vi "Main.vi"(11 "Module Admin":refnum<class "Delacor_lib_QMH_Cloneable Module Admin.lvclass">) -> ()   [LabVIEW 2020, in "FCR100.lvlib"]
doc: "This template is based off of the Queued Message Handler design pattern and the Queued Message Handler project template that ships with LabVIEW.\n\nThe main difference is that the queue is private to this module and communication between modules is performed via Broadcast and Request events.\n\nRequest events are wrapped in public API methods and are handled in the Event Handling Loop (EHL) of this VI. Any module can register for Broadcast events sent by this module. The EHL generates messages based on user interface actions.\n\nThe Message Handling Loop (MHL) processes messages generated by the EHL, or by other messages. The messages are string values, so new messages can be added easily to the Message Cases case structure in the MHL. Each message cluster can also provide an optional value for Message Data, which is a variant that can be converted to whatever message-specific data is required.\n_____\nBased on DQMH Project Template 6.1.0.94."
uses:
  FCR100.lvlib
  <vilib>/Delacor/Delacor QMH/Libraries/Cloneable Module Admin_class/Delacor_lib_QMH_Cloneable Module Admin.lvclass
  C:/Program Files (x86)/National Instruments/LabVIEW 2020/vi.lib/Delacor/Delacor QMH/Libraries/Module Admin_class/Delacor_lib_QMH_Module Admin.lvclass
  Support/Device state -- enum.ctl
  Support/Device states -- cluster.ctl
  Module Data--cluster.ctl
  Support/Device connection cluster -- cluster.ctl
  Support/HL data -- cluster.ctl
  <vilib>/Delacor/Delacor QMH/Libraries/Message Queue_class/Delacor_lib_QMH_Message Queue.lvclass/Delacor_lib_QMH_Message Queue.ctl
  <vilib>/Delacor/Delacor QMH/Libraries/Cloneable Module Admin_class/Delacor_lib_QMH_Cloneable Module Admin.lvclass/Delacor_lib_QMH_Cloneable Module Admin.ctl
  Stop Argument--cluster.ctl
  Connect with dialog Argument--cluster.ctl
  Connect with dialog (Reply Payload)--cluster.ctl
  Change configuration state Argument--cluster.ctl
  Change disable state Argument--cluster.ctl
  Search Home Argument--cluster.ctl
  Stop movement Argument--cluster.ctl
  Get state Argument--cluster.ctl
  Get state (Reply Payload)--cluster.ctl
  Set acceleration Argument--cluster.ctl
  Get acceleration Argument--cluster.ctl
  Get acceleration (Reply Payload)--cluster.ctl
  Set velocity Argument--cluster.ctl
  Get velocity Argument--cluster.ctl
  Get velocity (Reply Payload)--cluster.ctl
  Get ETA Argument--cluster.ctl
  Get ETA (Reply Payload)--cluster.ctl
  Move absolute Argument--cluster.ctl
  Move relative Argument--cluster.ctl
  Get current position Argument--cluster.ctl
  Get current position (Reply Payload)--cluster.ctl
  <vilib>/Delacor/Delacor QMH/Libraries/Module Admin_class/Delacor_lib_QMH_Module Admin.lvclass/Delacor_lib_QMH_Module Admin.ctl
  Reset controller Argument--cluster.ctl
  Find instruments Argument--cluster.ctl
  Find instruments (Reply Payload)--cluster.ctl
  Connect wihtout dialog Argument--cluster.ctl
  Disconnect Argument--cluster.ctl
  Continuously check state Argument--cluster.ctl
  Stop checking state Argument--cluster.ctl
  Configure simultaneous move Argument--cluster.ctl
  Get simultaneous move config Argument--cluster.ctl
  Get simultaneous move config (Reply Payload)--cluster.ctl
  Execute simultaneous move Argument--cluster.ctl
  <vilib>/Utility/miscctls.llb/LVPointTypeDef.ctl
  <vilib>/Instr/_visa.llb/VISA Flush IO Buffer Mask.ctl
  Support/Wake HL data -- cluster.ctl
  <vilib>/Delacor/Delacor QMH/Libraries/Message Queue_class/Delacor_lib_QMH_Enqueue Message (Array).vi
  <vilib>/Delacor/Delacor QMH/Libraries/Cloneable Module Admin_class/Delacor_lib_QMH_Get Module ID.vi
  <vilib>/Delacor/Delacor QMH/Libraries/Message Queue_class/Delacor_lib_QMH_Enqueue Message (Single).vi
  <vilib>/Delacor/Delacor QMH/Libraries/Module Admin_class/Delacor_lib_QMH_Get External Launch.vi
  <vilib>/Utility/error.llb/Error Cluster From Error Code.vi
  <vilib>/ErrorRing/Error Ring.xnode
  <vilib>/Delacor/Delacor QMH/Libraries/Message Queue_class/Delacor_lib_QMH_Message Queue.lvclass
panel:
  in  "Device state":T1=enum."Configuration"
  out "error out":errorcluster
  out "Status":string
  # "Other QMH Modules communicate with this Module via its Public API (wrappers for its Request Events).\n\nThis Module communicates with other Modules via its Broadcast Events.\nAny module that wants to get these messages, just registers for this module's Broadcast events."
  # "This template is for the Delacor Modified Queued Message Handler design pattern.\n\nSee the block diagram for more information on how to use this template."
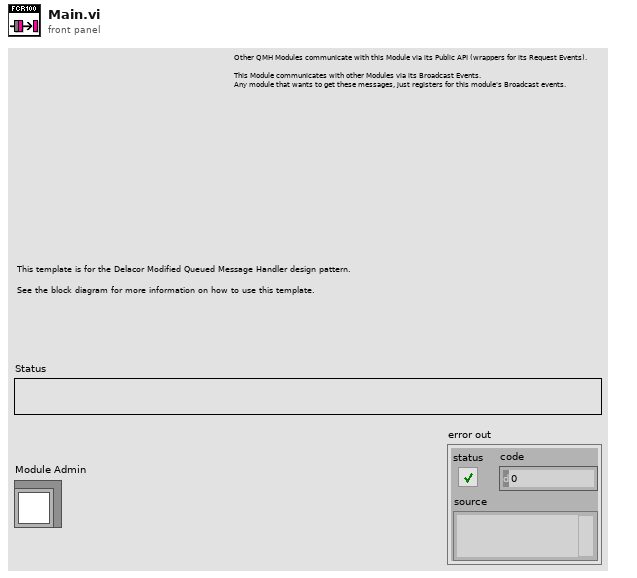
[diagram p1: front panel]
types:
  T1 = typedef "FCR100.lvlib/Device state -- enum.ctl" = enum16{"Not referenced", "Configuration", "Disable", "Ready", "Homing", "Motion"}
  T2 = typedef "FCR100.lvlib/Device states -- cluster.ctl" = cluster{"Address":u8, "Device state out":T1}
  T3 = typedef "FCR100.lvlib/Request Events--cluster.ctl" = cluster{"Stop Module":refnum<user-event>, "Show Panel":refnum<user-event>, "Hide Panel":refnum<user-event>, "Show Diagram":refnum<user-event>, "Get Module Execution Status":refnum<user-event>, "Connect with dialog":refnum<user-event>, "Change configuration state":refnum<user-event>, "Change disable state":refnum<user-event>, "Search Home":refnum<user-event>, "Stop movement":refnum<user-event>, "Get state":refnum<user-event>, "Set acceleration":refnum<user-event>, "Get acceleration":refnum<user-event>, "Set velocity":refnum<user-event>, "Get velocity":refnum<user-event>, "Get ETA":refnum<user-event>, "Move absolute":refnum<user-event>, "Move relative":refnum<user-event>, "Get current position":refnum<user-event>, "Reset controller":refnum<user-event>, "Find instruments":refnum<user-event>, "Connect wihtout dialog":refnum<user-event>, "Disconnect":refnum<user-event>, "Continuously check state":refnum<user-event>, "Stop checking state":refnum<user-event>, "Configure simultaneous move":refnum<user-event>, "Get simultaneous move config":refnum<user-event>, "Execute simultaneous move":refnum<user-event>}
  T4 = cluster{"Wake HL":refnum<user-event>, "Sleep HL":refnum<user-event>}
  T5 = typedef "FCR100.lvlib/HL data -- cluster.ctl" = cluster{"Instrument Channel":string, "Current state":T1, "Desired state":T1, "Address":u8, "Module ID":i32}
  T6 = typedef "FCR100.lvlib/Module Data--cluster.ctl" = cluster{"Status":string, "Device Connection Cluster":T7, "Connected?":bool, "Devices states":T1[], "Instrument Channel":string}
  T7 = typedef "Device connection cluster -- cluster.ctl" = cluster{"VISA resource name":refnum<visa-resource-name>, "Device name":string, "Controller address":i32, "error":errorcluster}
  T8 = enum32{"invalid lock state", "Not Locked", "Locked (No Password)", "Password-protected"}
  T9 = typedef "FCR100.lvlib/Stop Argument--cluster.ctl" = cluster{"Module ID":i32, "Origin":string, "Exit via Stop Module Req?":bool, "Wait for Module to stop?":bool}
  T10 = typedef "FCR100.lvlib/Connect with dialog Argument--cluster.ctl" = cluster{"Module ID":i32, "Baud Rate":u32, "Wait Notifier":refnum<notifier>, "wait for reply":bool}
  T11 = typedef "FCR100.lvlib/Change configuration state Argument--cluster.ctl" = cluster{"Module ID":i32, "Enter/(leave)":bool, "Address":u8}
  T12 = typedef "FCR100.lvlib/Change disable state Argument--cluster.ctl" = cluster{"Module ID":i32, "Enter/Leave":bool, "Address":u8}
  T13 = typedef "FCR100.lvlib/Search Home Argument--cluster.ctl" = cluster{"Module ID":i32, "Address":u8}
  T14 = typedef "FCR100.lvlib/Stop movement Argument--cluster.ctl" = cluster{"Module ID":i32, "Address":u8}
  T15 = typedef "FCR100.lvlib/Get state Argument--cluster.ctl" = cluster{"Module ID":i32, "Address":u8, "Wait Notifier":refnum<notifier>, "wait for reply":bool}
  T16 = typedef "FCR100.lvlib/Set acceleration Argument--cluster.ctl" = cluster{"Module ID":i32, "Address":u8, "Acceleration":u16}
  T17 = typedef "FCR100.lvlib/Get acceleration Argument--cluster.ctl" = cluster{"Module ID":i32, "Address":u8, "Wait Notifier":refnum<notifier>, "wait for reply":bool}
  T18 = typedef "FCR100.lvlib/Set velocity Argument--cluster.ctl" = cluster{"Module ID":i32, "Address":u8, "Velocity":u16}
  T19 = typedef "FCR100.lvlib/Get velocity Argument--cluster.ctl" = cluster{"Module ID":i32, "Address":u8, "Wait Notifier":refnum<notifier>, "wait for reply":bool}
  T20 = typedef "FCR100.lvlib/Get ETA Argument--cluster.ctl" = cluster{"Module ID":i32, "Address":u8, "Position":dbl, "Wait Notifier":refnum<notifier>, "wait for reply":bool}
  T21 = typedef "FCR100.lvlib/Move absolute Argument--cluster.ctl" = cluster{"Module ID":i32, "Address":u8, "Position":dbl}
  T22 = typedef "FCR100.lvlib/Move relative Argument--cluster.ctl" = cluster{"Module ID":i32, "Address":u8, "Position":dbl}
  T23 = typedef "FCR100.lvlib/Get current position Argument--cluster.ctl" = cluster{"Module ID":i32, "Address":u8, "Wait Notifier":refnum<notifier>, "wait for reply":bool}
  T24 = typedef "FCR100.lvlib/Reset controller Argument--cluster.ctl" = cluster{"Module ID":i32, "Address":u8}
  T25 = typedef "FCR100.lvlib/Find instruments Argument--cluster.ctl" = cluster{"Module ID":i32, "Wait Notifier":refnum<notifier>, "wait for reply":bool}
  T26 = typedef "FCR100.lvlib/Connect wihtout dialog Argument--cluster.ctl" = cluster{"Module ID":i32, "VISA resource":refnum<visa-resource-name>, "baud rate":u32}
  T27 = typedef "FCR100.lvlib/Disconnect Argument--cluster.ctl" = cluster{"Module ID":i32, "Boolean":bool}
  T28 = typedef "FCR100.lvlib/Continuously check state Argument--cluster.ctl" = cluster{"Module ID":i32, "Address":u8, "Desired state":T1, "Timeout":i32}
  T29 = typedef "FCR100.lvlib/Stop checking state Argument--cluster.ctl" = cluster{"Module ID":i32, "Address":u8}
  T30 = typedef "FCR100.lvlib/Configure simultaneous move Argument--cluster.ctl" = cluster{"Module ID":i32, "Address":u8, "Position":dbl}
  T31 = typedef "FCR100.lvlib/Get simultaneous move config Argument--cluster.ctl" = cluster{"Module ID":i32, "Address":u8, "Wait Notifier":refnum<notifier>, "wait for reply":bool}
  T32 = typedef "FCR100.lvlib/Execute simultaneous move Argument--cluster.ctl" = cluster{"Module ID":i32, "Boolean":bool}
  T33 = typedef "LVPointTypeDef.ctl" = cluster{"Horizontal":i16, "Vertical":i16}
  T34 = enum32{"Invalid", "Standard", "Closed", "Hidden", "Minimized", "Maximized"}
  T35 = typedef "FCR100.lvlib/Find instruments (Reply Payload)--cluster.ctl" = cluster{"error":errorcluster, "Resource Names":string[], "Interface Names":string[]}
  T36 = typedef "FCR100.lvlib/Connect with dialog (Reply Payload)--cluster.ctl" = cluster{"Connected?":bool, "error":errorcluster}
  T37 = typedef "FCR100.lvlib/Get state (Reply Payload)--cluster.ctl" = cluster{"Device state":T1, "error":errorcluster}
  T38 = typedef "FCR100.lvlib/Get acceleration (Reply Payload)--cluster.ctl" = cluster{"Acceleration":u16, "error":errorcluster}
  T39 = typedef "FCR100.lvlib/Get velocity (Reply Payload)--cluster.ctl" = cluster{"Velocity":u16, "error":errorcluster}
  T40 = typedef "FCR100.lvlib/Get ETA (Reply Payload)--cluster.ctl" = cluster{"ETA":dbl, "error":errorcluster}
  T41 = typedef "FCR100.lvlib/Get current position (Reply Payload)--cluster.ctl" = cluster{"Position":dbl, "error":errorcluster}
  T42 = typedef "FCR100.lvlib/Wake HL data -- cluster.ctl" = cluster{"Timeout":i32, "Instrument Channel":string, "Address":u8, "Current state":T1, "Desired state":T1, "Module ID":i32}
  T43 = typedef "FCR100.lvlib/Get simultaneous move config (Reply Payload)--cluster.ctl" = cluster{"Response":string, "error":errorcluster}
  T44 = cluster{"VISA resource name":refnum<visa-resource-name>, "Device name":string, "Controller address":i32, "error":errorcluster}
  T45 = typedef "VISA Flush IO Buffer Mask.ctl" = u16
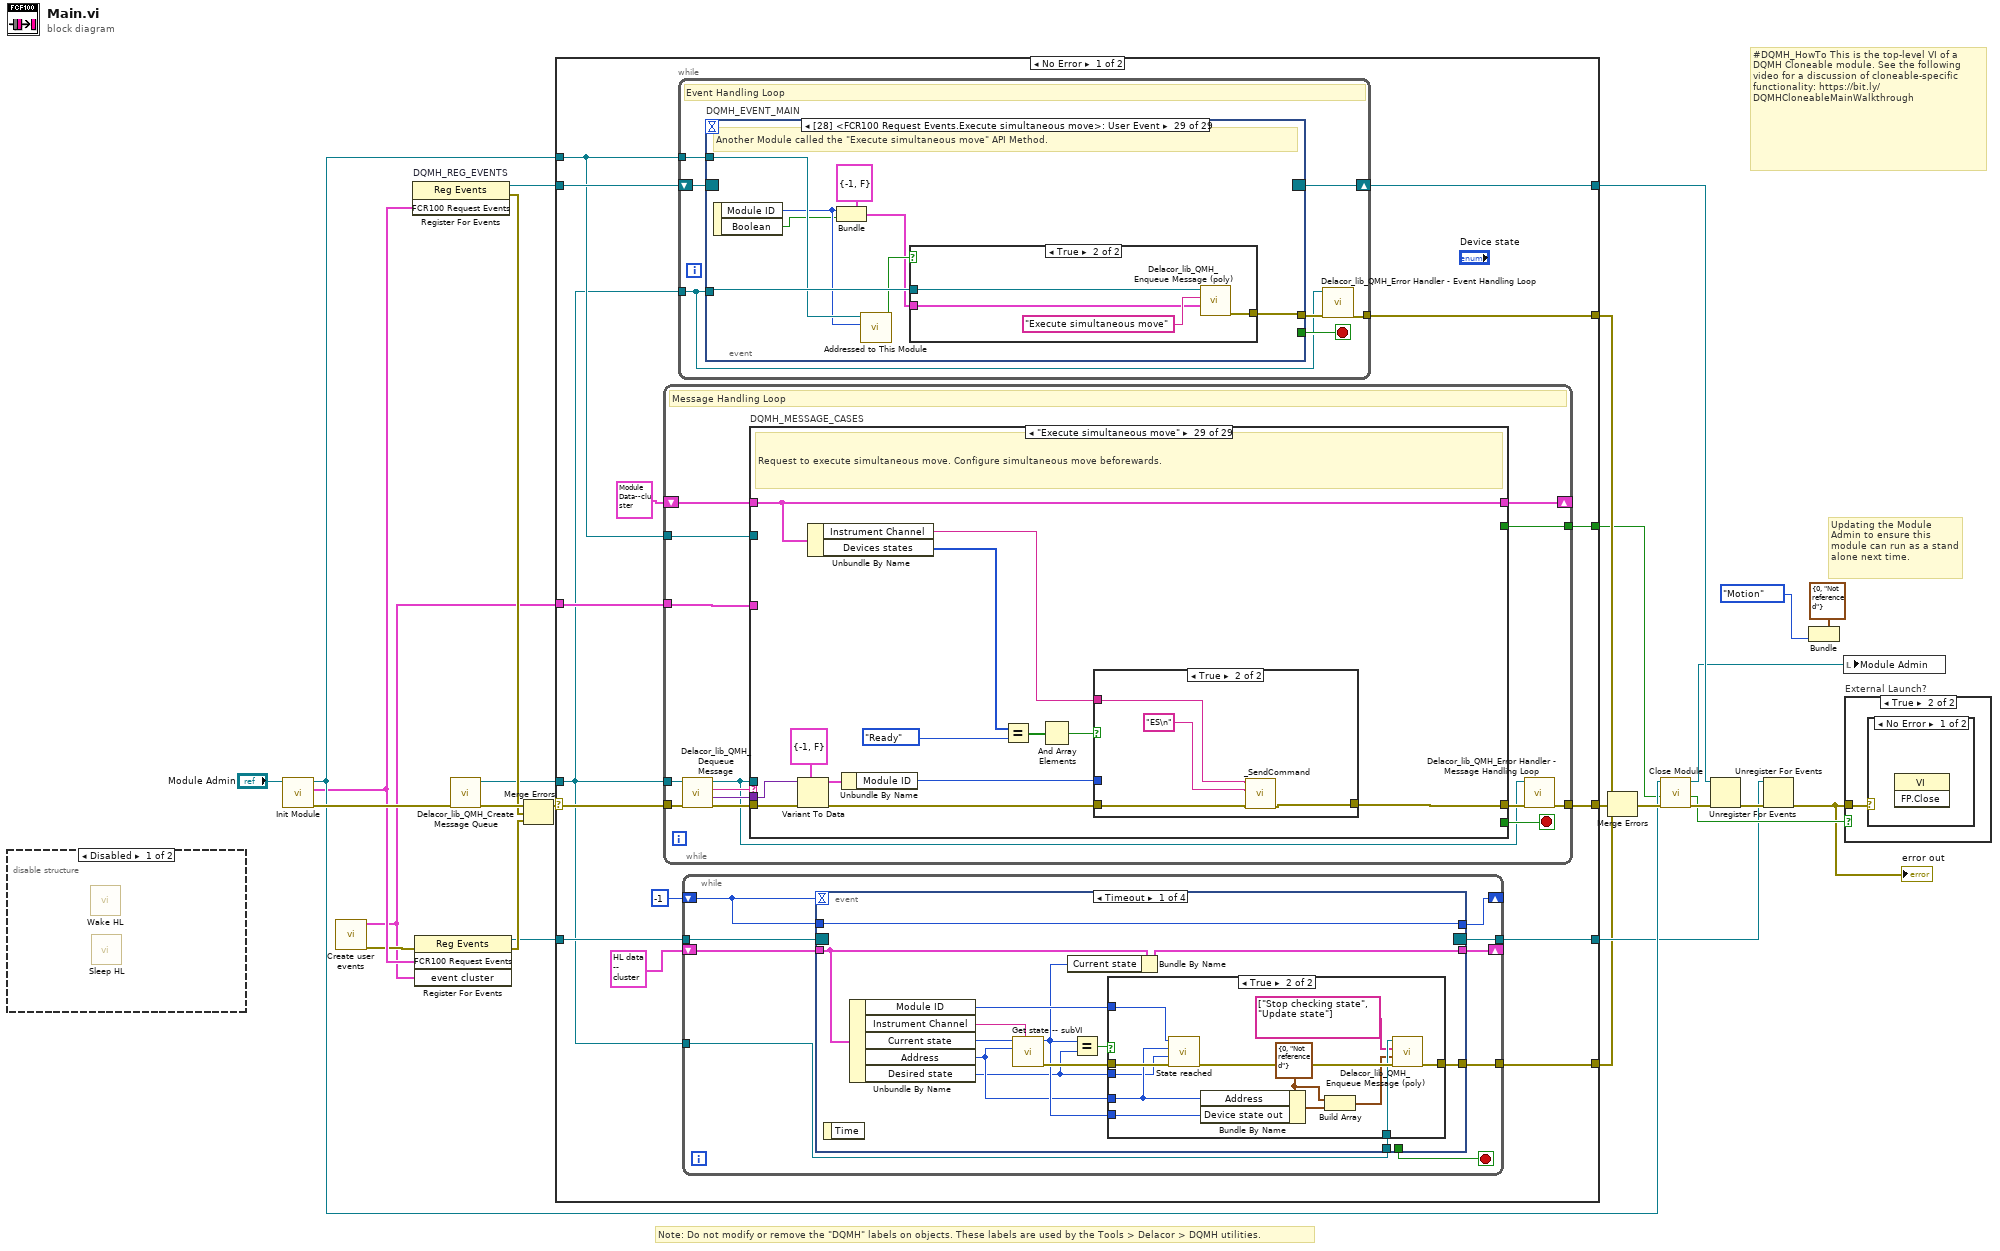
[diagram p0: block diagram]
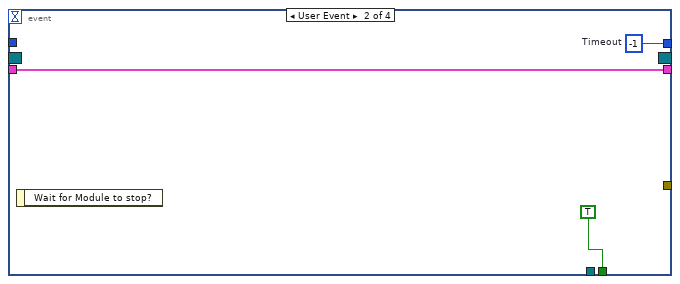
[diagram p4: hidden frame]
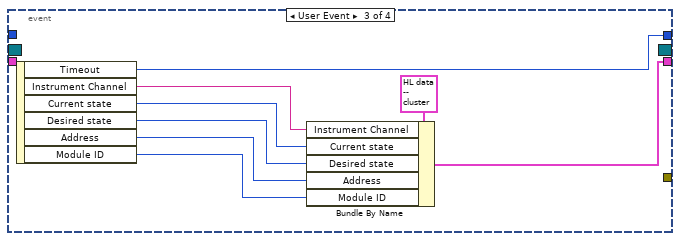
[diagram p5: hidden frame]
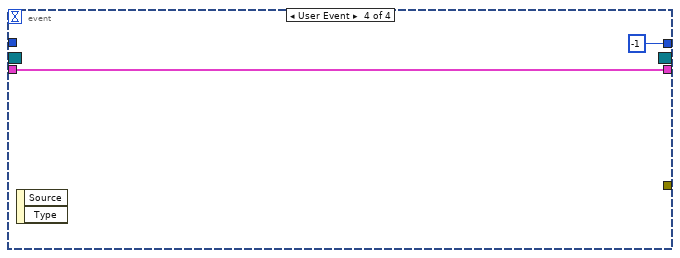
[diagram p6: hidden frame]
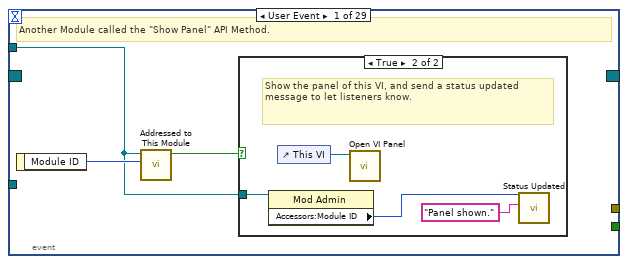
[diagram p7: hidden frame]
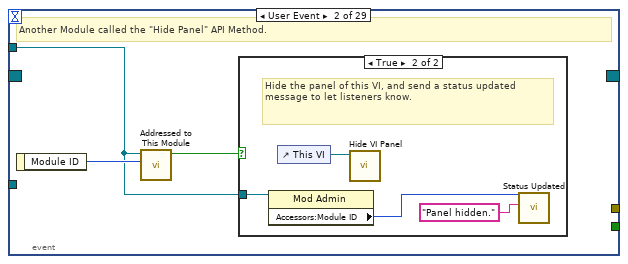
[diagram p9: hidden frame]
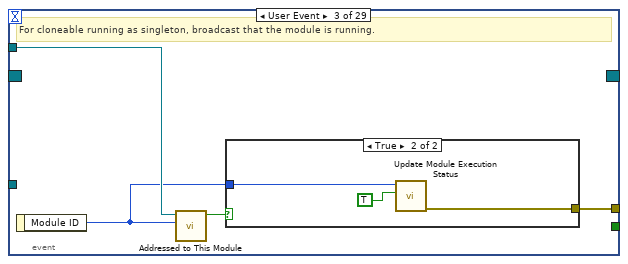
[diagram p11: hidden frame]
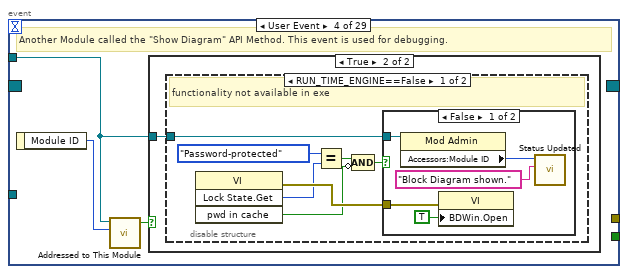
[diagram p13: hidden frame]
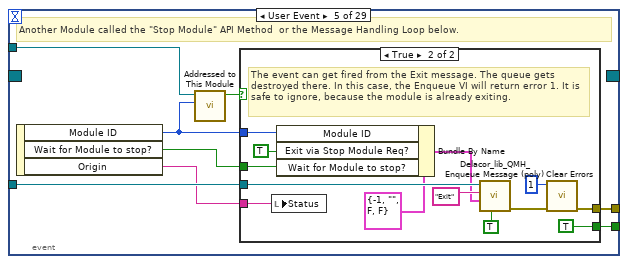
[diagram p17: hidden frame]
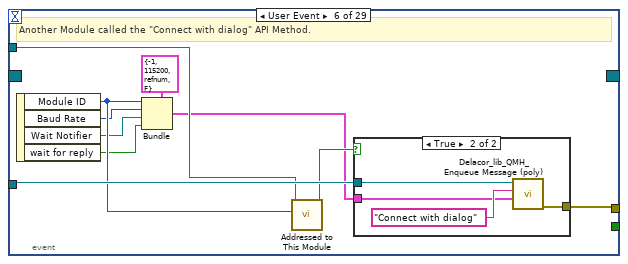
[diagram p19: hidden frame]
diagram:
  # "#DQMH_HowTo This is the top-level VI of a DQMH Cloneable module. See the following video for a discussion of cloneable-specific functionality: https://bit.ly/DQMHCloneableMainWalkthrough"
  # "Note: Do not modify or remove the \"DQMH\" labels on objects. These labels are used by the Tools > Delacor > DQMH utilities."
  # "Updating the Module Admin to ensure this module can run as a stand alone next time."
  n1 = disable-structure shown="Disabled" {
    frame Disabled {
      n2 = call "Wake HL.vi"() -> ()  [unwired: 11 in, 1 out]
      n3 = call "Sleep HL.vi"() -> ()  [unwired: 11 in, 1 out]
    }
    frame Enabled {
    }
  }
  n4 = call "Init Module.vi"("Cloneable Module Admin in"="Module Admin") -> ("error out"=w24:errorcluster, "FCR100 Request Events"=w11:T3, "Cloneable Module Admin out"=w15:refnum<class "Delacor_lib_QMH_Cloneable Module Admin.lvclass">)  [unwired: 8 in]
  n5 = call "Create user events.vi"() -> ("error out"=w10:errorcluster, "event cluster"=w7:T4)  [unwired: 10 in]
  n6 = register-events "DQMH_REG_EVENTS"(w11) -> (reference out=w18:refnum<event-registration>, error out=w20:errorcluster)  [unwired: 2 in]
  n7 = register-events(error in=w10, w11, w7) -> (reference out=w8:refnum<event-registration>, error out=w9:errorcluster)  [unwired: 1 in]
  n8 = call <vilib>:"Delacor_lib_QMH_Create Message Queue.vi"("error in"=w24) -> ("error out"=w22:errorcluster, "Message Queue"=w17:refnum<class "Delacor_lib_QMH_Message Queue.lvclass">)  [unwired: 9 in]
  n9 = Merge Errors(w22, w20, w9) -> (w21:errorcluster)
  n10 = case shown="No Error" w21 {
    selector: w21 -> [w40 w1397]
    tunnel: [w42 w1396] -> w25
    tunnel: [w39 w1404] -> w19
    tunnel: w18 -> [w37 w1404]
    tunnel: w17 -> [w31 w1395]
    tunnel: [w41 _] -> w26
    tunnel: w15 -> [w36 w1400]
    tunnel: [w35 _] -> w13
    tunnel: w8 -> [w34 w1394]
    tunnel: w7 -> [w33 _]
    tunnel: [w32 w1394] -> w4
    tunnel: [w28 _] -> w3
    frame No Error {
      n11 = while {
        tunnel: w31 -> [w471]
        shift-right: [w475] -> _
        shift-left: T6 {"Status"="", "Device Connection Cluster"={"VISA resource name"="", "Device name"="", "Controller address"=0, "error"={"status"=FALSE, "code"=0, "source"=""}}, "Connected?"=FALSE, "Devices states"=[], "Instrument Channel"="GPIB/0:4,0"} ("Data Cluster") -> [w476]
        tunnel: w40 -> [w479]
        tunnel: [w477] -> w42
        tunnel: w36 -> [w469]
        tunnel: [w468] -> w35
        tunnel: w33 -> [w467]
        stop <- w474 stop-if-true
        # "Message Handling Loop"
        n12 = call-dynamic "Delacor_lib_QMH_Dequeue Message.vi"("error in"=w479, "Message Queue in"=w471) -> ("error out"=w478:errorcluster, "Message Data"=w472:variant, "Message"=w473:string, "Message Queue out"=w470:refnum<class "Delacor_lib_QMH_Message Queue.lvclass">)  [unwired: 6 in]
        n13 = case "DQMH_MESSAGE_CASES" shown="\"Execute simultaneous move\"" w473 {
          selector: w473 -> [_ _ _ _ _ _ _ _ _ _ _ _ _ _ _ _ _ _ _ _ _ _ _ w1258 _ _ _ _ _]
          tunnel: w470 -> [_ _ _ _ _ _ w661 w707 w746 w792 w834 _ _ _ _ _ w1066 w1115 _ _ _ w1223 w1248 _ _ _ _ _ _]
          tunnel: w478 -> [w499 w515 w530 w605 w639 w651 w669 w715 w755 w800 w846 w864 w906 w945 w987 w1031 w1077 w1126 w1176 w1204 w1221 w1232 w1254 w1260 w1287 w1296 w1310 w1348 w1385]
          tunnel: [w497 w505 w520 w596 w627 w649 w663 w710 w750 w794 w837 w859 w897 w939 w978 w1022 w1072 w1121 w1167 w1199 w1221 w1228 w1251 w1261 w1282 w1290 w1305 w1339 w1380] -> w480
          tunnel: w476 -> [w491 w514 w523 w595 w624 w647 w662 w708 w747 w793 w829 w858 w895 w941 w977 w1020 w1071 w1118 w1166 w1195 w1220 w1227 w1247 w1259 w1281 w1295 w1303 w1338 w1379]
          tunnel: [w490 w514 w522 w594 w622 w648 w662 w708 w747 w793 w828 w858 w895 w941 w977 w1020 w1071 w1118 w1166 w1192 w1220 w1227 w1247 w1259 w1281 w1295 w1303 w1338 w1379] -> w475
          tunnel: [_ _ _ _ _ _ _ _ _ _ _ _ _ _ _ _ _ _ _ _ _ _ w1246 _ _ _ _ _ _] -> w474
          tunnel: w472 -> [_ w512 w529 w603 w638 w650 w668 w714 w754 w799 w844 w863 w904 w944 w985 w1029 w1076 w1125 w1174 w1203 _ w1226 w1244 _ w1286 w1294 w1309 w1346 w1384]
          tunnel: w469 -> [w486 _ _ _ _ _ _ _ _ _ _ _ _ _ _ _ _ _ _ _ _ w1225 w1240 w1256 _ _ _ _ _]
          tunnel: [_ _ _ _ _ _ _ _ _ _ _ _ _ _ _ _ _ _ _ _ _ _ w1242 _ _ _ _ _ _] -> w468
          tunnel: w467 -> [_ _ _ _ _ _ _ _ _ _ _ _ _ _ _ _ _ _ _ _ _ _ _ _ w1280 w1289 _ _ _]
          frame "Initialize" {
            w481 = T1[] [] items=["Not referenced", "Configuration", "Disable", "Ready", "Homing", "Motion"] ("Devices states")
            w489 = TRUE  # Initialized?
            w483 = "Initial Message" ("Initial Message")
            # "Initialize - Any operation that needs to be done before the module can receive messages. Synchronize Caller Events.vi will inform Start Module.vi that the module has launched and is ready to receive messages. Module Did Init.vi will broadcast that the module initialized."
            n14 = call "Synchronize Caller Events.vi"("error in (no error)"=w499, "Module Admin"=w486) -> ("error out"=w498:errorcluster, "Module Admin out"=w485:refnum<class "Delacor_lib_QMH_Cloneable Module Admin.lvclass">)  [unwired: 8 in]
            n15 = property on="Property Node" class="Mod Admin"(reference=w485) -> ("Accessors:Module ID"=w488:i32, "Accessors:External Launch"=w487:bool)  [unwired: 1 in, 2 out]
            n16 = call "Module Name--constant.vi"("Module ID"=w488) -> ("Module Name"=w482:string)  [unwired: 10 in]
            n17 = property on="Property Node" class="VI"("Front Panel.Title"=w482) -> (reference out=w496:refnum<vi>, error out=w501:errorcluster)  [unwired: 2 in]
            n18 = Select(t=T34."Hidden" ("State"), s=w487, f=T34."Standard" ("State")) -> (s? t:f=w492:T34)
            n19 = invoke on="Invoke Node" class="VI" method="FP.Open"(reference=w496, error in=w501, "State"=w492) -> (reference out=w495:refnum<vi>, error out=w500:errorcluster)  [unwired: 2 in, 3 out]
            n20 = property on="Pane" class="Pane"("Origin"=T33 {"Horizontal"=0, "Vertical"=0}) -> ()  [unwired: 2 in, 2 out]
            n21 = invoke on="Invoke Node" class="VI" method="FP.Center"(reference=w495, error in=w500) -> ()  [unwired: 1 in, 3 out]
            n22 = Bundle By Name(cluster=w491, "Devices states"=w481, "Status"=w483) -> (w490:T6)
            n23 = call "Module Did Init.vi"("error in (no error)"=w498, "Initialized?"=w489, "Origin"=w482, "Module ID"=w488) -> ("error out"=w497:errorcluster)  [unwired: 7 in]
            "Status" <- w483
          }
          frame "Find instruments" {
            # "Request to find connected instruments."
            n24 = Variant To Data(error in=w515, type=T25 {"Module ID"=-1, "Wait Notifier"=refnum, "wait for reply"=FALSE} ("Find instruments Argument"), Variant=w512) -> (data=w510:T25, error out=w513:errorcluster)
            n25 = Unbundle By Name(w510) -> ("Wait Notifier"=w509:refnum<notifier>, "wait for reply"=w508:bool)  [unwired: 1 out]
            n26 = call "FindInstrument.vi"() -> ("error out"=w504:errorcluster, "Found Interface Names"=w502:string[], "Found Resource Names"=w503:string[])  [unwired: 9 in]
            n27 = Merge Errors(w513, w504) -> (w505:errorcluster)
            n28 = Bundle By Name(cluster=T35 {"error"={"status"=FALSE, "code"=0, "source"=""}, "Resource Names"=[], "Interface Names"=[]} ("Find instruments (Reply Payload)"), "Resource Names"=w503, "Interface Names"=w502, "error"=w504) -> (w507:T35)
            n29 = case shown="True" w508 {
              tunnel: w509 -> [_ w517]
              tunnel: w507 -> [_ w516]
              frame False {
              }
              frame True {
                n30 = Send Notification(notification=w516, notifier=w517) -> ()  [unwired: 1 in, 2 out]
              }
            }
          }
          frame "Connect wihtout dialog" {
            # "Request to connect to device without using dialog."
            n31 = Variant To Data(error in=w530, type=T26 {"Module ID"=-1, "VISA resource"="", "baud rate"=115200} ("Connect wihtout dialog Argument"), Variant=w529) -> (data=w527:T26, error out=w526:errorcluster)
            n32 = Unbundle By Name(w527) -> ("VISA resource"=w525:refnum<visa-resource-name>, "baud rate"=w524:u32, "Module ID"=w519:i32)
            n33 = VISA Open(error in (no error)=w526, VISA resource name=w525) -> (VISA resource name=w518:refnum<visa-resource-name>, error out=w521:errorcluster)  [unwired: 3 in]
            n34 = case shown="No Error" w521 {
              selector: w521 -> [w535 w567 w570 w586]
              tunnel: w524 -> [w541 _ _ _]
              tunnel: w523 -> [w537 w565 w577 w584]
              tunnel: [w536 w565 w577 w584] -> w522
              tunnel: [w534 w561 w573 w580] -> w520
              tunnel: w519 -> [w533 w560 w572 w579]
              tunnel: w518 -> [w532 _ _ _]
              frame No Error {
                n35 = property class="Instr"(reference=w532) -> ("Intf Inst Name"=w531:string)  [unwired: 1 in, 2 out]
                n36 = call "_Parse Instrument Channel.vi"("Instrument Channel"=w531) -> ("T - GPIB, F - RS232"=w540:bool, "Hardware Address"=w538:i32, "Instrument Address"=w539:i16, "Valid String"=w542:bool)  [unwired: 6 in, 1 out]
                n37 = case shown="False" w542 {
                  tunnel: w538 -> [_ w558]
                  tunnel: w540 -> [_ w555]
                  tunnel: w539 -> [_ w557]
                  tunnel: w541 -> [_ w556]
                  tunnel: w537 -> [w547 w554]
                  tunnel: [w547 w553] -> w536
                  tunnel: w535 -> [w546 w551]
                  tunnel: [w545 w550] -> w534
                  tunnel: w533 -> [w544 w549]
                  frame False {
                    # "Invalid string"
                    n38 = call "Connection failed.vi"("error in"=w546, "Connected?"=FALSE, "Module ID"=w544) -> ("error out"=w545:errorcluster)  [unwired: 8 in]
                  }
                  frame True {
                    # "Valid string"
                    n39 = call "_Create Instrument Channel.vi"("Baud Rate (921600 - USB)"=w556, "COM Port (1)"=w558, "GPIB Primary Address (4)"=w557, "(F), T - GPIB, F - RS232"=w555) -> ("Instrument Channel out"=w552:string)  [unwired: 5 in, 2 out]
                    n40 = Bundle By Name(cluster=w554, "Instrument Channel"=w552) -> (w553:T6)
                    n41 = call "Device connected.vi"("error in"=w551, "Connected?"=TRUE, "Module ID"=w549) -> ("error out"=w550:errorcluster)  [unwired: 8 in]
                  }
                }
              }
              frame Error {
                n42 = call <vilib>:"Clear Errors.vi"("error in (no error)"=w567, "specific error code to clear (0: all)"=-1073807346) -> ("error out"=w564:errorcluster)  [unwired: 4 in, 1 out]
                n43 = call "Connection failed.vi"("error in"=w564, "Connected?"=FALSE, "Module ID"=w560) -> ("error out"=w562:errorcluster)  [unwired: 8 in]
                n44 = call "Status Updated.vi"("error in (no error)"=w562, "Status"="Could not find any device connected do port.", "Module ID"=w560) -> ("error out"=w561:errorcluster)  [unwired: 8 in]
              }
              frame Default {
                n45 = call <vilib>:"Clear Errors.vi"("error in (no error)"=w570) -> ("error out"=w576:errorcluster)  [unwired: 5 in, 1 out]
                n46 = Unbundle By Name(w570) -> ("code"=w569:i32)
                n47 = call "Connection failed.vi"("error in"=w576, "Connected?"=FALSE, "Module ID"=w572) -> ("error out"=w574:errorcluster)  [unwired: 8 in]
                n48 = Format Into String(format string="Unknown error. Error code: %d." ("Status"), w569) -> (resulting string=w568:string)  [unwired: 2 in, 1 out]
                n49 = call "Status Updated.vi"("error in (no error)"=w574, "Status"=w568, "Module ID"=w572) -> ("error out"=w573:errorcluster)  [unwired: 8 in]
              }
              frame Error {
                n50 = call <vilib>:"Clear Errors.vi"("error in (no error)"=w586, "specific error code to clear (0: all)"=-1073807343) -> ("error out"=w583:errorcluster)  [unwired: 4 in, 1 out]
                n51 = call "Connection failed.vi"("error in"=w583, "Connected?"=FALSE, "Module ID"=w579) -> ("error out"=w581:errorcluster)  [unwired: 8 in]
                n52 = call "Status Updated.vi"("error in (no error)"=w581, "Status"="Device has been disconnected.", "Module ID"=w579) -> ("error out"=w580:errorcluster)  [unwired: 8 in]
              }
            }
          }
          frame "Connect with dialog" {
            # "Request to launch Newport connection dialog and try to connect to selected device."
            n53 = Variant To Data(error in=w605, type=T10 {"Module ID"=-1, "Baud Rate"=115200, "Wait Notifier"=refnum, "wait for reply"=FALSE} ("Connect with dialog Argument"), Variant=w603) -> (data=w601:T10, error out=w604:errorcluster)
            n54 = Unbundle By Name(w601) -> ("Baud Rate"=w589:u32, "Module ID"=w588:i32, "Wait Notifier"=w600:refnum<notifier>, "wait for reply"=w599:bool)
            n55 = call "Connect Newport Instrument.vi"("Baud Rate (115200 - USB)"=w589) -> ("error (duplicate)"=w591:errorcluster, "Connected"=w592:bool, "VISA resource name (duplicate)"=w587:refnum<visa-resource-name>, "Device Connection Cluster"=w593:T44)  [unwired: 6 in, 1 out]
            n56 = case shown="False" w592 {
              selector: w592 -> [w606 w613]
              tunnel: w595 -> [w611 w619]
              tunnel: [w610 w618] -> w594
              tunnel: w593 -> [_ w615]
              tunnel: w591 -> [w609 w617]
              tunnel: [w608 w616] -> w590
              tunnel: w588 -> [w607 w614]
              tunnel: w587 -> [_ w612]
              frame False {
                # "Device not connected"
                n57 = Bundle By Name(cluster=w611, "Connected?"=w606) -> (w610:T6)
                n58 = call "Connection failed.vi"("error in"=w609, "Connected?"=w606, "Module ID"=w607) -> ("error out"=w608:errorcluster)  [unwired: 8 in]
              }
              frame True {
                # "Device connected"
                n59 = Bundle By Name(cluster=w619, "Device Connection Cluster"=w615, "Instrument Channel"=w612, "Connected?"=w613) -> (w618:T6)
                n60 = call "Device connected.vi"("error in"=w617, "Connected?"=w613, "Module ID"=w614) -> ("error out"=w616:errorcluster)  [unwired: 8 in]
              }
            }
            n61 = Bundle By Name(cluster=T36 {"Connected?"=FALSE, "error"={"status"=FALSE, "code"=0, "source"=""}} ("Connect with dialog (Reply Payload)"), "Connected?"=w592, "error"=w590) -> (w598:T36)
            n62 = case shown="True" w599 {
              tunnel: w600 -> [_ w621]
              tunnel: w598 -> [_ w620]
              frame False {
              }
              frame True {
                n63 = Send Notification(notification=w620, notifier=w621) -> ()  [unwired: 1 in, 2 out]
              }
            }
            n64 = Merge Errors(w604, w590) -> (w596:errorcluster)
          }
          frame "Disconnect" {
            w625 = FALSE  # Connected?
            w630 = T45 128 items=["Flush Receive Buffer"=16, "Write Transmit Buffer to Device"=32, "Flush Receive Buffer (No I/O)"=64, "Flush Transmit Buffer"=128] ("Mask")
            w631 = T45 64 items=["Flush Receive Buffer"=16, "Write Transmit Buffer to Device"=32, "Flush Receive Buffer (No I/O)"=64, "Flush Transmit Buffer"=128] ("Mask")
            # "Request to close connection with a device."
            n65 = Variant To Data(error in=w639, type=T27 {"Module ID"=-1, "Boolean"=FALSE} ("Disconnect Argument"), Variant=w638) -> (data=w636:T27, error out=w634:errorcluster)
            n66 = Unbundle By Name(w624) -> ("Instrument Channel"=w635:string)
            n67 = Unbundle By Name(w636) -> ("Module ID"=w626:i32)
            n68 = Or(x=w631, y=w630) -> (x .or. y?=w629:T45)
            n69 = VISA Flush I/O Buffer(VISA resource name=w635, mask (16)=w629, error in (no error)=w634) -> (VISA resource name out=w632:refnum<visa-resource-name>, error out=w633:errorcluster)
            n70 = VISA Close(VISA resource name=w632, error in (no error)=w633) -> (error out=w628:errorcluster)
            n71 = Bundle By Name(cluster=w624, "Connected?"=FALSE) -> (w622:T6)
            n72 = call "Device disconnected.vi"("error in"=w628, "Connected?"=w625, "Module ID"=w626) -> ("error out"=w627:errorcluster)  [unwired: 8 in]
          }
          frame "Update state" {
            # "Changes internally the current state of the controller."
            n73 = Variant To Data(error in=w651, type=T2 {"Address"=0, "Device state out"=enum."Not referenced"}, Variant=w650) -> (data=w646:T2, error out=w649:errorcluster)
            n74 = Unbundle By Name(w647) -> ("Devices states"=w643:T1[])
            n75 = Unbundle(w646) -> ("Address"=w644:u8, "Device state out"=w641:T1)
            n76 = Decrement(x=w644) -> (x-1=w642:u8)
            n77 = in-place {
              in-place-border: w641 -> [w652]
              n78 = in-place-array #1(w643, w642) -> ()  [unwired: 1 out]
              n79 = in-place-array #1(w652) -> (w640:T1[])  [unwired: 1 out]
            }
            n80 = Bundle By Name(cluster=w647, "Devices states"=w640) -> (w648:T6)
          }
          frame "Change configuration state" {
            # "Request to enter/leave configuration state."
            n81 = Unbundle By Name(w662) -> ("Devices states"=w655:T1[], "Instrument Channel"=w659:string)
            n82 = Variant To Data(error in=w669, type=T11 {"Module ID"=-1, "Enter/(leave)"=FALSE, "Address"=0} ("Change configuration state Argument"), Variant=w668) -> (data=w666:T11, error out=w664:errorcluster)
            n83 = Unbundle By Name(w666) -> ("Module ID"=w657:i32, "Address"=w654:u8, "Enter/(leave)"=w665:bool)
            n84 = Decrement(x=w654) -> (x-1=w653:u8)
            n85 = Index Array(array=w655, index=w653) -> (element=w656:T1)
            n86 = Not Equal To 0?(x=w654) -> (x != 0?=w658:bool)
            n87 = case shown="True" w658 {
              tunnel: w665 -> [_ w679]
              tunnel: w656 -> [_ w678]
              tunnel: w661 -> [_ w677]
              tunnel: [w672 w676] -> w660
              tunnel: w654 -> [_ w675]
              tunnel: w659 -> [_ w674]
              tunnel: w657 -> [w670 w673]
              frame False {
                # "Address is zero. Broadcast not allowed for this command."
                n88 = call "Status Updated.vi"("Status"="Current operation does not admit broadcast. Select a controller address different than 0.", "Module ID"=w670) -> ("error out"=w672:errorcluster)  [unwired: 9 in]
              }
              frame True {
                # "Address not zero. Execute command."
                n89 = case shown="\"Not referenced\", \"Configuration\"" w678 {
                  selector: w678 -> [w682 _]
                  tunnel: w679 -> [_ w692]
                  tunnel: w677 -> [_ w699]
                  tunnel: [w686 w698] -> w676
                  tunnel: w675 -> [_ w688]
                  tunnel: w674 -> [_ w695]
                  tunnel: w673 -> [w685 _]
                  frame Default {
                    # "Current state does not admit this command."
                    n90 = property on="Device state" class="Enum (strict)"() -> ("Strings []"=w683:string[])  [unwired: 2 in, 2 out]
                    n91 = Index Array(array=w683, index=w682) -> (element=w681:string)
                    n92 = Format Into String(format string="Change in configuration state only allowed in Not referenced or Configuration states. Current state: %s." ("Status"), w681) -> (resulting string=w680:string)  [unwired: 2 in, 1 out]
                    n93 = call "Status Updated.vi"("Status"=w680, "Module ID"=w685) -> ("error out"=w686:errorcluster)  [unwired: 9 in]
                  }
                  frame "Not referenced", "Configuration" {
                    n94 = Boolean To (0,1)(Boolean=w692) -> (0, 1=w693:i16)
                    n95 = Format Into String(format string="%dPW%d", w688, w693) -> (resulting string=w691:string)  [unwired: 2 in, 1 out]
                    n96 = Select(t=Device_state_--_enum."Configuration" ("Device state"), s=w692, f=Device_state_--_enum."Not referenced") -> (s? t:f=w689:T1)
                    n97 = call "_SendCommand.vi"("Command"=w691, "Instrument Channel"=w695) -> ("error out"=w696:errorcluster)  [unwired: 8 in, 1 out]
                    n98 = Bundle(cluster=T2 {"Address"=0, "Device state out"=enum."Not referenced"}, "Address"=w688, "Device state out"=w689) -> (w687:T2)
                    n99 = call-poly <vilib>:"Delacor_lib_QMH_Enqueue Message (poly).vi"("error in"=w696, "Message Data"=w687, "Message"="Update state", "Message Queue in"=w699) -> ("error out"=w698:errorcluster)  [unwired: 6 in, 1 out]
                  }
                }
              }
            }
            n100 = Merge Errors(w664, w660) -> (w663:errorcluster)
          }
          frame "Change disable state" {
            # "Request to modify DISABLE state. Set to enter, clear to leave. (xxMMnn)"
            n101 = Unbundle By Name(w708) -> ("Devices states"=w705:T1[])
            n102 = Variant To Data(error in=w715, type=T12 {"Module ID"=-1, "Enter/Leave"=FALSE, "Address"=0} ("Change disable state Argument"), Variant=w714) -> (data=w712:T12, error out=w711:errorcluster)
            n103 = Unbundle By Name(w712) -> ("Module ID"=w706:i32, "Address"=w704:u8, "Enter/Leave"=w709:bool)
            n104 = Decrement(x=w704) -> (x-1=w703:u8)
            n105 = Index Array(array=w705, index=w703) -> (element=w702:T1)
            n106 = case shown="\"Disable\", \"Ready\"" w702 {
              selector: w702 -> [w716 _]
              tunnel: w711 -> [w721 w740]
              tunnel: [w720 w728] -> w710
              tunnel: w704 -> [_ w725]
              tunnel: w709 -> [_ w736]
              tunnel: w708 -> [_ w734]
              tunnel: w707 -> [_ w729]
              tunnel: w706 -> [w717 _]
              frame Default {
                n107 = property on="Device state" class="Enum (strict)"() -> ("Strings []"=w719:string[])  [unwired: 2 in, 2 out]
                n108 = Index Array(array=w719, index=w716) -> (element=w718:string)
                n109 = Format Into String(format string="Change in disable state only allowed in Ready or Disabled states. Current state: %s." ("Status"), w718) -> (resulting string=w722:string)  [unwired: 2 in, 1 out]
                n110 = call "Status Updated.vi"("error in (no error)"=w721, "Status"=w722, "Module ID"=w717) -> ("error out"=w720:errorcluster)  [unwired: 8 in]
              }
              frame "Disable", "Ready" {
                n111 = Unbundle By Name(w734) -> ("Instrument Channel"=w735:string)
                n112 = Boolean To (0,1)(Boolean=w736) -> (0, 1=w738:i16)
                n113 = Format Into String(format string="%0.2dMM%0.1d\n", w725, w738) -> (resulting string=w737:string)  [unwired: 2 in, 1 out]
                n114 = Select(t=Device_state_--_enum."Ready" ("Device state"), s=w736, f=Device_state_--_enum."Disable" ("Device state")) -> (s? t:f=w726:T1)
                n115 = call "_SendCommand.vi"("error in"=w740, "Command"=w737, "Instrument Channel"=w735) -> ("error out"=w731:errorcluster)  [unwired: 7 in, 1 out]
                n116 = Bundle(cluster=T2 {"Address"=0, "Device state out"=enum."Not referenced"}, "Address"=w725, "Device state out"=w726) -> (w724:T2)
                n117 = call-poly <vilib>:"Delacor_lib_QMH_Enqueue Message (poly).vi"("error in"=w731, "Message Data"=w724, "Message"="Update state", "Message Queue in"=w729) -> ("error out"=w728:errorcluster)  [unwired: 6 in, 1 out]
              }
            }
          }
          frame "Search Home" {
            # "Request to execute home search (xxOR, {Not referenced})"
            n118 = Variant To Data(error in=w755, type=T13 {"Module ID"=-1, "Address"=0} ("Search Home Argument"), Variant=w754) -> (data=w752:T13, error out=w751:errorcluster)
            n119 = Unbundle By Name(w747) -> ("Instrument Channel"=w749:string, "Devices states"=w744:T1[])
            n120 = Unbundle By Name(w752) -> ("Module ID"=w745:i32, "Address"=w742:u8)
            n121 = Decrement(x=w742) -> (x-1=w741:u8)
            n122 = Not Equal To 0?(x=w742) -> (x != 0?=w748:bool)
            n123 = Index Array(array=w744, index=w741) -> (element=w743:T1)
            n124 = case shown="True" w748 {
              tunnel: w751 -> [w758 w766]
              tunnel: [w757 w765] -> w750
              tunnel: w749 -> [_ w764]
              tunnel: w742 -> [_ w763]
              tunnel: w746 -> [_ w762]
              tunnel: w745 -> [w756 w761]
              tunnel: w743 -> [_ w760]
              frame False {
                # "Broadcast not allowed for this command. Use address different from 0."
                n125 = call "Status Updated.vi"("error in (no error)"=w758, "Status"="Broadcast not allowed for this command. Use an address different from 0.", "Module ID"=w756) -> ("error out"=w757:errorcluster)  [unwired: 8 in]
              }
              frame True {
                # "Address is not zero. Execute command."
                n126 = case shown="\"Not referenced\"" w760 {
                  selector: w760 -> [_ w780]
                  tunnel: w766 -> [w778 w784]
                  tunnel: [w772 w783] -> w765
                  tunnel: w764 -> [w777 _]
                  tunnel: w763 -> [w768 _]
                  tunnel: w762 -> [w771 _]
                  tunnel: w761 -> [_ w779]
                  frame "Not referenced" {
                    n127 = Format Into String(format string="%dOR\n", w768) -> (resulting string=w775:string)  [unwired: 2 in, 1 out]
                    n128 = call "_SendCommand.vi"("error in"=w778, "Command"=w775, "Instrument Channel"=w777) -> ("error out"=w773:errorcluster)  [unwired: 7 in, 1 out]
                    n129 = Bundle(cluster=T2 {"Address"=0, "Device state out"=enum."Not referenced"}, "Address"=w768, "Device state out"=Device_state_--_enum."Homing" ("Device state")) -> (w767:T2)
                    n130 = call-poly <vilib>:"Delacor_lib_QMH_Enqueue Message (poly).vi"("error in"=w773, "Message Data"=w767, "Message"="Update state", "Message Queue in"=w771) -> ("error out"=w772:errorcluster)  [unwired: 6 in, 1 out]
                  }
                  frame Default {
                    n131 = property on="Device state" class="Enum (strict)"() -> ("Strings []"=w782:string[])  [unwired: 2 in, 2 out]
                    n132 = Index Array(array=w782, index=w780) -> (element=w781:string)
                    n133 = Format Into String(format string="Seach home only allowed in Not referenced state. Current state: %s." ("Status"), w781) -> (resulting string=w785:string)  [unwired: 2 in, 1 out]
                    n134 = call "Status Updated.vi"("error in (no error)"=w784, "Status"=w785, "Module ID"=w779) -> ("error out"=w783:errorcluster)  [unwired: 8 in]
                  }
                }
              }
            }
          }
          frame "Stop movement" {
            # "Request to stop movement of a single or multilple motors (xxST)"
            n135 = Unbundle By Name(w793) -> ("Instrument Channel"=w795:string, "Devices states"=w790:T1[])
            n136 = Variant To Data(error in=w800, type=T14 {"Module ID"=-1, "Address"=0} ("Stop movement Argument"), Variant=w799) -> (data=w797:T14, error out=w796:errorcluster)
            n137 = Unbundle By Name(w797) -> ("Module ID"=w791:i32, "Address"=w788:u8)
            n138 = Decrement(x=w788) -> (x-1=w787:u8)
            n139 = Index Array(array=w790, index=w787) -> (element=w789:T1)
            n140 = case shown="\"Homing\", \"Motion\"" w789 {
              selector: w789 -> [_ w815]
              tunnel: w796 -> [w803 w819]
              tunnel: w795 -> [_ w818]
              tunnel: [w802 w810] -> w794
              tunnel: w788 -> [_ w806]
              tunnel: w792 -> [_ w809]
              tunnel: w791 -> [w801 _]
              frame Default {
                n141 = call "Status Updated.vi"("error in (no error)"=w803, "Status"="Controller not in motion. Cannot stop.", "Module ID"=w801) -> ("error out"=w802:errorcluster)  [unwired: 8 in]
              }
              frame "Homing", "Motion" {
                n142 = Equal?(x=w815, y=Device_state_--_enum."Motion" ("Device state")) -> (x = y?=w816:bool)
                n143 = Format Into String(format string="%dST\n", w806) -> (resulting string=w821:string)  [unwired: 2 in, 1 out]
                n144 = Select(t=Device_state_--_enum."Ready" ("Device state"), s=w816, f=Device_state_--_enum."Not referenced" ("Device state")) -> (s? t:f=w807:T1)
                n145 = call "_SendCommand.vi"("error in"=w819, "Command"=w821, "Instrument Channel"=w818) -> ("error out"=w811:errorcluster)  [unwired: 7 in, 1 out]
                n146 = Bundle(cluster=T2 {"Address"=0, "Device state out"=enum."Not referenced"}, "Address"=w806, "Device state out"=w807) -> (w805:T2)
                n147 = call-poly <vilib>:"Delacor_lib_QMH_Enqueue Message (poly).vi"("error in"=w811, "Message Data"=w805, "Message"="Update state", "Message Queue in"=w809) -> ("error out"=w810:errorcluster)  [unwired: 6 in, 1 out]
              }
            }
          }
          frame "Get state" {
            # "Request to get error and controller state (xxTS)."
            n148 = Variant To Data(error in=w846, type=T15 {"Module ID"=-1, "Address"=0, "Wait Notifier"=refnum, "wait for reply"=FALSE} ("Get state Argument"), Variant=w844) -> (data=w842:T15, error out=w845:errorcluster)
            n149 = Unbundle By Name(w829) -> ("Instrument Channel"=w833:string, "Devices states"=w825:T1[])
            n150 = Unbundle By Name(w842) -> ("Address"=w827:u8, "Wait Notifier"=w841:refnum<notifier>, "wait for reply"=w840:bool)  [unwired: 1 out]
            n151 = Decrement(x=w827) -> (x-1=w824:u8)
            n152 = Index Array(array=w825, index=w824) -> (element=w832:T1)
            n153 = call "Get state -- subVI.vi"("Instrument Channel"=w833, "Address"=w827, "Device state in"=w832) -> ("error out"=w836:errorcluster, "Device state out"=w823:T1)  [unwired: 7 in]
            n154 = in-place {
              in-place-border: w823 -> [w847]
              n155 = in-place-array #2(w825, w824) -> ()  [unwired: 1 out]
              n156 = in-place-array #2(w847) -> (w822:T1[])  [unwired: 1 out]
            }
            n157 = Bundle(cluster=T2 {"Address"=0, "Device state out"=enum."Not referenced"}, "Address"=w827, "Device state out"=w823) -> (w830:T2)
            n158 = call-poly <vilib>:"Delacor_lib_QMH_Enqueue Message (poly).vi"("error in"=w836, "Message Data"=w830, "Message"="Update state", "Message Queue in"=w834) -> ("error out"=w835:errorcluster)  [unwired: 6 in, 1 out]
            n159 = Bundle By Name(cluster=w829, "Devices states"=w822) -> (w828:T6)
            n160 = Bundle By Name(cluster=T37 {"Device state"=enum."Not referenced", "error"={"status"=FALSE, "code"=0, "source"=""}} ("Get state (Reply Payload)"), "Device state"=w823, "error"=w835) -> (w839:T37)
            n161 = case shown="True" w840 {
              tunnel: w841 -> [_ w849]
              tunnel: w839 -> [_ w848]
              frame False {
              }
              frame True {
                n162 = Send Notification(notification=w848, notifier=w849) -> ()  [unwired: 1 in, 2 out]
              }
            }
            n163 = Merge Errors(w845, w835) -> (w837:errorcluster)
          }
          frame "Set acceleration" {
            (unwired) Device_state_--_enum."Configuration" ("Device state")
            # "Request to change the acceleration of the device (xxACnn)"
            n164 = Variant To Data(error in=w864, type=T16 {"Module ID"=-1, "Address"=0, "Acceleration"=0} ("Set acceleration Argument"), Variant=w863) -> (data=w861:T16, error out=w860:errorcluster)
            n165 = Unbundle By Name(w858) -> ("Instrument Channel"=w857:string, "Devices states"=w853:T1[])
            n166 = Unbundle By Name(w861) -> ("Address"=w851:u8, "Acceleration"=w856:u16, "Module ID"=w854:i32)
            n167 = Decrement(x=w851) -> (x-1=w850:u8)
            n168 = Index Array(array=w853, index=w850) -> (element=w852:T1)
            n169 = Not Equal To 0?(x=w851) -> (x != 0?=w855:bool)
            n170 = case shown="True" w855 {
              tunnel: w860 -> [w868 w875]
              tunnel: [w867 w874] -> w859
              tunnel: w852 -> [_ w873]
              tunnel: w857 -> [_ w872]
              tunnel: w856 -> [_ w871]
              tunnel: w851 -> [_ w870]
              tunnel: w854 -> [w865 w869]
              frame False {
                # "Address is 0. Broadcast not allowed."
                n171 = call "Status Updated.vi"("error in (no error)"=w868, "Status"="Broadcast not allowed for this command. Use an address different from 0.", "Module ID"=w865) -> ("error out"=w867:errorcluster)  [unwired: 8 in]
              }
              frame True {
                # "Address not zero. Execute command."
                n172 = case shown="\"Configuration\"..\"Ready\"" w873 {
                  tunnel: w875 -> [w878 w884]
                  tunnel: [w877 w883] -> w874
                  tunnel: w872 -> [_ w882]
                  tunnel: w871 -> [_ w881]
                  tunnel: w870 -> [_ w880]
                  tunnel: w869 -> [w876 _]
                  frame Default {
                    n173 = call "Status Updated.vi"("error in (no error)"=w878, "Status"="Cannot set acceleration while in motion or not referenced. Stop the controller motion and try again.", "Module ID"=w876) -> ("error out"=w877:errorcluster)  [unwired: 8 in]
                  }
                  frame "Configuration".."Ready" {
                    n174 = Format Into String(format string="%dAC%d\n", w880, w881) -> (resulting string=w886:string)  [unwired: 2 in, 1 out]
                    n175 = call "_SendCommand.vi"("error in"=w884, "Command"=w886, "Instrument Channel"=w882) -> ("error out"=w883:errorcluster)  [unwired: 7 in, 1 out]
                  }
                }
              }
            }
          }
          frame "Get acceleration" {
            # "Request to get current acceleration (xxAC?)."
            n176 = Unbundle By Name(w895) -> ("Instrument Channel"=w894:string, "Devices states"=w889:T1[])
            n177 = Variant To Data(error in=w906, type=T17 {"Module ID"=-1, "Address"=0, "Wait Notifier"=refnum, "wait for reply"=FALSE} ("Get acceleration Argument"), Variant=w904) -> (data=w902:T17, error out=w905:errorcluster)
            n178 = Unbundle By Name(w902) -> ("Address"=w888:u8, "Module ID"=w891:i32, "Wait Notifier"=w901:refnum<notifier>, "wait for reply"=w900:bool)
            n179 = Not Equal To 0?(x=w888) -> (x != 0?=w893:bool)
            n180 = Decrement(x=w888) -> (x-1=w887:u8)
            n181 = Index Array(array=w889, index=w887) -> (element=w890:T1)
            n182 = case shown="True" w893 {
              tunnel: [w909 w915] -> w896
              tunnel: w890 -> [_ w914]
              tunnel: w894 -> [_ w913]
              tunnel: w888 -> [_ w912]
              tunnel: [_ w911] -> w892
              tunnel: w891 -> [w907 w910]
              frame False {
                # "Address is 0. Broadcast not allowed."
                n183 = call "Status Updated.vi"("Status"="Broadcast not allowed for this command. Use an address different from 0.", "Module ID"=w907) -> ("error out"=w909:errorcluster)  [unwired: 9 in]
              }
              frame True {
                # "Address not zero. Execute command."
                n184 = case shown="\"Configuration\"..\"Ready\"" w914 {
                  tunnel: [w918 w926] -> w915
                  tunnel: w913 -> [_ w925]
                  tunnel: w912 -> [_ w927]
                  tunnel: [_ w920] -> w911
                  tunnel: w910 -> [w916 _]
                  frame Default {
                    n185 = call "Status Updated.vi"("Status"="Cannot get velocity while in motion. Stop the controller motion and try again.", "Module ID"=w916) -> ("error out"=w918:errorcluster)  [unwired: 9 in]
                  }
                  frame "Configuration".."Ready" {
                    w919 = u16 0  # U16
                    n186 = Format Into String(format string="%dAC?\n", w927) -> (resulting string=w924:string)  [unwired: 2 in, 1 out]
                    n187 = call "_QueryCommand.vi"("Command"=w924, "Instrument Channel in"=w925) -> ("error out"=w926:errorcluster, "Response"=w923:string)  [unwired: 7 in, 1 out]
                    n188 = Match Pattern(string=w923, regular expression="AC") -> (after substring=w921:string)  [unwired: 1 in, 3 out]
                    n189 = Decimal String To Number(string=w921, default (0L)=w919) -> (number=w920:u16)  [unwired: 1 in, 1 out]
                  }
                }
              }
            }
            n190 = Bundle By Name(cluster=T38 {"Acceleration"=0, "error"={"status"=FALSE, "code"=0, "source"=""}} ("Get acceleration (Reply Payload)"), "Acceleration"=w892, "error"=w896) -> (w899:T38)
            n191 = Merge Errors(w905, w896) -> (w897:errorcluster)
            n192 = case shown="True" w900 {
              tunnel: w901 -> [_ w930]
              tunnel: w899 -> [_ w929]
              frame False {
              }
              frame True {
                n193 = Send Notification(notification=w929, notifier=w930) -> ()  [unwired: 1 in, 2 out]
              }
            }
          }
          frame "Set velocity" {
            # "Request to set a new velocity (xxVAnn)."
            n194 = Variant To Data(error in=w945, type=T18 {"Module ID"=-1, "Address"=0, "Velocity"=0} ("Set velocity Argument"), Variant=w944) -> (data=w942:T18, error out=w940:errorcluster)
            n195 = Unbundle By Name(w941) -> ("Instrument Channel"=w936:string, "Devices states"=w934:T1[])
            n196 = Unbundle By Name(w942) -> ("Address"=w932:u8, "Velocity"=w938:u16, "Module ID"=w935:i32)
            n197 = Decrement(x=w932) -> (x-1=w931:u8)
            n198 = Index Array(array=w934, index=w931) -> (element=w933:T1)
            n199 = Not Equal To 0?(x=w932) -> (x != 0?=w937:bool)
            n200 = case shown="True" w937 {
              tunnel: w940 -> [w949 w956]
              tunnel: [w948 w955] -> w939
              tunnel: w933 -> [_ w954]
              tunnel: w936 -> [_ w953]
              tunnel: w938 -> [_ w952]
              tunnel: w932 -> [_ w951]
              tunnel: w935 -> [w947 w950]
              frame False {
                # "Address is 0. Broadcast not allowed."
                n201 = call "Status Updated.vi"("error in (no error)"=w949, "Status"="Broadcast not allowed for this command. Use an address different than 0.", "Module ID"=w947) -> ("error out"=w948:errorcluster)  [unwired: 8 in]
              }
              frame True {
                # "Address not zero. Execute command."
                n202 = case shown="\"Configuration\"..\"Ready\"" w954 {
                  tunnel: w956 -> [w960 w965]
                  tunnel: [w959 w964] -> w955
                  tunnel: w953 -> [_ w963]
                  tunnel: w952 -> [_ w962]
                  tunnel: w951 -> [_ w961]
                  tunnel: w950 -> [w958 _]
                  frame Default {
                    n203 = call "Status Updated.vi"("error in (no error)"=w960, "Status"="Cannot set velocity while in motion or not referenced. Stop the controller motion and try again.", "Module ID"=w958) -> ("error out"=w959:errorcluster)  [unwired: 8 in]
                  }
                  frame "Configuration".."Ready" {
                    n204 = Format Into String(format string="%dVA%d\n", w961, w962) -> (resulting string=w967:string)  [unwired: 2 in, 1 out]
                    n205 = call "_SendCommand.vi"("error in"=w965, "Command"=w967, "Instrument Channel"=w963) -> ("error out"=w964:errorcluster)  [unwired: 7 in, 1 out]
                  }
                }
              }
            }
          }
          frame "Get velocity" {
            # "Request to get the current velocity of the specified device (xxVA?)."
            n206 = Variant To Data(error in=w987, type=T19 {"Module ID"=-1, "Address"=0, "Wait Notifier"=refnum, "wait for reply"=FALSE} ("Get velocity Argument"), Variant=w985) -> (data=w983:T19, error out=w986:errorcluster)
            n207 = Unbundle By Name(w977) -> ("Instrument Channel"=w976:string, "Devices states"=w970:T1[])
            n208 = Unbundle By Name(w983) -> ("Address"=w969:u8, "Module ID"=w972:i32, "Wait Notifier"=w982:refnum<notifier>, "wait for reply"=w981:bool)
            n209 = Decrement(x=w969) -> (x-1=w968:u8)
            n210 = Index Array(array=w970, index=w968) -> (element=w971:T1)
            n211 = Not Equal To 0?(x=w969) -> (x != 0?=w975:bool)
            n212 = case shown="True" w975 {
              tunnel: [w989 w995] -> w973
              tunnel: w971 -> [_ w994]
              tunnel: w976 -> [_ w993]
              tunnel: [_ w992] -> w974
              tunnel: w972 -> [w988 _]
              tunnel: w969 -> [_ w991]
              frame False {
                # "Address is 0. Broadcast not allowed."
                n213 = call "Status Updated.vi"("Status"="Cannot set acceleration while in motion. Stop the controller motion and try again.", "Module ID"=w988) -> ("error out"=w989:errorcluster)  [unwired: 9 in]
              }
              frame True {
                # "Address not zero. Execute command."
                n214 = case shown="\"Configuration\"..\"Ready\"" w994 {
                  tunnel: [w996 w1007] -> w995
                  tunnel: w993 -> [_ w1006]
                  tunnel: [_ w1001] -> w992
                  tunnel: w991 -> [w997 w999]
                  frame Default {
                    n215 = call "Status Updated.vi"("Status"="Cannot  get velocity while in motion. Stop the controller motion and try again.", "Module ID"=w997) -> ("error out"=w996:errorcluster)  [unwired: 9 in]
                  }
                  frame "Configuration".."Ready" {
                    w1000 = u16 0  # U16
                    n216 = Format Into String(format string="%dVA?\n", w999) -> (resulting string=w1005:string)  [unwired: 2 in, 1 out]
                    n217 = call "_QueryCommand.vi"("Command"=w1005, "Instrument Channel in"=w1006) -> ("error out"=w1007:errorcluster, "Response"=w1004:string)  [unwired: 7 in, 1 out]
                    n218 = Match Pattern(string=w1004, regular expression="VA") -> (after substring=w1002:string)  [unwired: 1 in, 3 out]
                    n219 = Decimal String To Number(string=w1002, default (0L)=w1000) -> (number=w1001:u16)  [unwired: 1 in, 1 out]
                  }
                }
              }
            }
            n220 = Bundle By Name(cluster=T39 {"Velocity"=0, "error"={"status"=FALSE, "code"=0, "source"=""}} ("Get velocity (Reply Payload)"), "Velocity"=w974, "error"=w973) -> (w980:T39)
            n221 = Merge Errors(w986, w973) -> (w978:errorcluster)
            n222 = case shown="True" w981 {
              tunnel: w982 -> [_ w1010]
              tunnel: w980 -> [_ w1009]
              frame False {
              }
              frame True {
                n223 = Send Notification(notification=w1009, notifier=w1010) -> ()  [unwired: 1 in, 2 out]
              }
            }
          }
          frame "Get ETA" {
            # "Request to get estimated duration in seconds of relative move (xxPTnn, {Disabled, Ready, Motion})"
            n224 = Variant To Data(error in=w1031, type=T20 {"Module ID"=-1, "Address"=0, "Position"=0.0, "Wait Notifier"=refnum, "wait for reply"=FALSE} ("Get ETA Argument"), Variant=w1029) -> (data=w1027:T20, error out=w1030:errorcluster)
            n225 = Unbundle By Name(w1020) -> ("Instrument Channel"=w1019:string, "Devices states"=w1014:T1[])
            n226 = Unbundle By Name(w1027) -> ("Address"=w1012:u8, "Position"=w1017:dbl, "Module ID"=w1015:i32, "Wait Notifier"=w1026:refnum<notifier>, "wait for reply"=w1025:bool)
            n227 = Decrement(x=w1012) -> (x-1=w1011:u8)
            n228 = Not Equal To 0?(x=w1012) -> (x != 0?=w1021:bool)
            n229 = Index Array(array=w1014, index=w1011) -> (element=w1013:T1)
            n230 = case shown="True" w1021 {
              tunnel: [w1034 w1041] -> w1016
              tunnel: w1013 -> [_ w1040]
              tunnel: w1019 -> [_ w1039]
              tunnel: w1012 -> [_ w1038]
              tunnel: [_ w1037] -> w1018
              tunnel: w1017 -> [_ w1036]
              tunnel: w1015 -> [w1033 w1035]
              frame False {
                # "Address is 0. Broadcast not allowed."
                n231 = call "Status Updated.vi"("Status"="Broadcast not allowed for this command. Use an address other than 0.", "Module ID"=w1033) -> ("error out"=w1034:errorcluster)  [unwired: 9 in]
              }
              frame True {
                # "Address not zero. Execute command."
                n232 = case shown="\"Disable\", \"Ready\", \"Motion\"" w1040 {
                  selector: w1040 -> [w1042 _]
                  tunnel: [w1048 w1057] -> w1041
                  tunnel: w1039 -> [_ w1056]
                  tunnel: w1038 -> [_ w1058]
                  tunnel: [_ w1051] -> w1037
                  tunnel: w1036 -> [_ w1049]
                  tunnel: w1035 -> [w1047 _]
                  frame Default {
                    n233 = property on="Device state" class="Enum (strict)"() -> ("Strings []"=w1045:string[])  [unwired: 2 in, 2 out]
                    n234 = Index Array(array=w1045, index=w1042) -> (element=w1044:string)
                    n235 = Format Into String(format string="Cannot get estimated time while on Not referenced or Configuration state. Current state: %s." ("Status"), w1044) -> (resulting string=w1043:string)  [unwired: 2 in, 1 out]
                    n236 = call "Status Updated.vi"("Status"=w1043, "Module ID"=w1047) -> ("error out"=w1048:errorcluster)  [unwired: 9 in]
                  }
                  frame "Disable", "Ready", "Motion" {
                    w1050 = 0.0  # DBL
                    n237 = Format Into String(format string="%dPT%0.1f\n", w1058, w1049) -> (resulting string=w1055:string)  [unwired: 2 in, 1 out]
                    n238 = call "_QueryCommand.vi"("Command"=w1055, "Instrument Channel in"=w1056) -> ("error out"=w1057:errorcluster, "Response"=w1054:string)  [unwired: 7 in, 1 out]
                    n239 = Match Pattern(string=w1054, regular expression="PT") -> (after substring=w1052:string)  [unwired: 1 in, 3 out]
                    n240 = Decimal String To Number(string=w1052, default (0L)=w1050) -> (number=w1051:dbl)  [unwired: 1 in, 1 out]
                  }
                }
              }
            }
            n241 = Bundle By Name(cluster=T40 {"ETA"=0.0, "error"={"status"=FALSE, "code"=0, "source"=""}} ("Get ETA (Reply Payload)"), "ETA"=w1018, "error"=w1016) -> (w1024:T40)
            n242 = Merge Errors(w1030, w1016) -> (w1022:errorcluster)
            n243 = case shown="True" w1025 {
              tunnel: w1026 -> [_ w1061]
              tunnel: w1024 -> [_ w1060]
              frame False {
              }
              frame True {
                n244 = Send Notification(notification=w1060, notifier=w1061) -> ()  [unwired: 1 in, 2 out]
              }
            }
          }
          frame "Move absolute" {
            # "Request to execute an absolute movement (xxPAnn, {Ready})"
            n245 = Unbundle By Name(w1071) -> ("Instrument Channel"=w1070:string, "Devices states"=w1065:T1[])
            n246 = Variant To Data(error in=w1077, type=T21 {"Module ID"=-1, "Address"=0, "Position"=0.0} ("Move absolute Argument"), Variant=w1076) -> (data=w1074:T21, error out=w1073:errorcluster)
            n247 = Unbundle By Name(w1074) -> ("Address"=w1063:u8, "Position"=w1068:dbl, "Module ID"=w1067:i32)
            n248 = Decrement(x=w1063) -> (x-1=w1062:u8)
            n249 = Index Array(array=w1065, index=w1062) -> (element=w1064:T1)
            n250 = Not Equal To 0?(x=w1063) -> (x != 0?=w1069:bool)
            n251 = case shown="True" w1069 {
              tunnel: w1073 -> [w1080 w1089]
              tunnel: [w1079 w1088] -> w1072
              tunnel: w1064 -> [_ w1087]
              tunnel: w1070 -> [_ w1086]
              tunnel: w1068 -> [_ w1085]
              tunnel: w1063 -> [_ w1084]
              tunnel: w1067 -> [w1078 w1083]
              tunnel: w1066 -> [_ w1082]
              frame False {
                # "Address is 0. Broadcast not allowed."
                n252 = call "Status Updated.vi"("error in (no error)"=w1080, "Status"="Broadcast not allowed for this command. Use an address other than 0.", "Module ID"=w1078) -> ("error out"=w1079:errorcluster)  [unwired: 8 in]
              }
              frame True {
                # "Address not zero. Execute command."
                n253 = case shown="Default" w1087 {
                  selector: w1087 -> [w1090 _]
                  tunnel: w1089 -> [w1097 w1108]
                  tunnel: [w1096 w1104] -> w1088
                  tunnel: w1086 -> [_ w1107]
                  tunnel: w1085 -> [_ w1106]
                  tunnel: w1084 -> [_ w1099]
                  tunnel: w1083 -> [w1095 _]
                  tunnel: w1082 -> [_ w1103]
                  frame Default {
                    n254 = property on="Device state" class="Enum (strict)"() -> ("Strings []"=w1094:string[])  [unwired: 2 in, 2 out]
                    n255 = Index Array(array=w1094, index=w1090) -> (element=w1091:string)
                    n256 = Format Into String(format string="Absolute move only allowed in Ready state. Current state: %s" ("Status"), w1091) -> (resulting string=w1092:string)  [unwired: 2 in, 1 out]
                    n257 = call "Status Updated.vi"("error in (no error)"=w1097, "Status"=w1092, "Module ID"=w1095) -> ("error out"=w1096:errorcluster)  [unwired: 8 in]
                  }
                  frame "Ready" {
                    n258 = Format Into String(format string="%dPA%0.3f\n", w1099, w1106) -> (resulting string=w1110:string)  [unwired: 2 in, 1 out]
                    n259 = call "_SendCommand.vi"("error in"=w1108, "Command"=w1110, "Instrument Channel"=w1107) -> ("error out"=w1105:errorcluster)  [unwired: 7 in, 1 out]
                    n260 = Bundle(cluster=T2 {"Address"=0, "Device state out"=enum."Not referenced"}, "Address"=w1099, "Device state out"=Device_state_--_enum."Motion" ("Device state")) -> (w1098:T2)
                    n261 = call-poly <vilib>:"Delacor_lib_QMH_Enqueue Message (poly).vi"("error in"=w1105, "Message Data"=w1098, "Message"="Update state", "Message Queue in"=w1103) -> ("error out"=w1104:errorcluster)  [unwired: 6 in, 1 out]
                  }
                }
              }
            }
          }
          frame "Move relative" {
            # "Request to execute a relative movement (PR, {Ready})"
            n262 = Unbundle By Name(w1118) -> ("Instrument Channel"=w1117:string, "Devices states"=w1114:T1[])
            n263 = Variant To Data(error in=w1126, type=T22 {"Module ID"=-1, "Address"=0, "Position"=0.0} ("Move relative Argument"), Variant=w1125) -> (data=w1123:T22, error out=w1122:errorcluster)
            n264 = Unbundle By Name(w1123) -> ("Address"=w1112:u8, "Position"=w1120:dbl, "Module ID"=w1116:i32)
            n265 = Decrement(x=w1112) -> (x-1=w1111:u8)
            n266 = Not Equal To 0?(x=w1112) -> (x != 0?=w1119:bool)
            n267 = Index Array(array=w1114, index=w1111) -> (element=w1113:T1)
            n268 = case shown="True" w1119 {
              tunnel: w1122 -> [w1129 w1138]
              tunnel: [w1128 w1137] -> w1121
              tunnel: w1113 -> [_ w1136]
              tunnel: w1117 -> [_ w1135]
              tunnel: w1120 -> [_ w1134]
              tunnel: w1112 -> [_ w1133]
              tunnel: w1116 -> [w1127 w1132]
              tunnel: w1115 -> [_ w1131]
              frame False {
                # "Address is 0. Broadcast not allowed."
                n269 = call "Status Updated.vi"("error in (no error)"=w1129, "Status"="Broadcast not allowed for this command. Use an address other than 0.", "Module ID"=w1127) -> ("error out"=w1128:errorcluster)  [unwired: 8 in]
              }
              frame True {
                # "Address not zero. Execute command."
                n270 = case shown="Default" w1136 {
                  selector: w1136 -> [w1142 _]
                  tunnel: w1138 -> [w1146 w1157]
                  tunnel: [w1145 w1151] -> w1137
                  tunnel: w1135 -> [_ w1156]
                  tunnel: w1134 -> [_ w1155]
                  tunnel: w1133 -> [_ w1148]
                  tunnel: w1132 -> [w1144 _]
                  tunnel: w1131 -> [_ w1152]
                  frame Default {
                    n271 = property on="Device state" class="Enum (strict)"() -> ("Strings []"=w1143:string[])  [unwired: 2 in, 2 out]
                    n272 = Index Array(array=w1143, index=w1142) -> (element=w1140:string)
                    n273 = Format Into String(format string="Relative movement only allowed in Ready state. Current state: %s." ("Status"), w1140) -> (resulting string=w1139:string)  [unwired: 2 in, 1 out]
                    n274 = call "Status Updated.vi"("error in (no error)"=w1146, "Status"=w1139, "Module ID"=w1144) -> ("error out"=w1145:errorcluster)  [unwired: 8 in]
                  }
                  frame "Ready" {
                    n275 = Format Into String(format string="%dPR%0.3f\n", w1148, w1155) -> (resulting string=w1159:string)  [unwired: 2 in, 1 out]
                    n276 = call "_SendCommand.vi"("error in"=w1157, "Command"=w1159, "Instrument Channel"=w1156) -> ("error out"=w1153:errorcluster)  [unwired: 7 in, 1 out]
                    n277 = Bundle(cluster=T2 {"Address"=0, "Device state out"=enum."Not referenced"}, "Address"=w1148, "Device state out"=Device_state_--_enum."Motion" ("Device state")) -> (w1147:T2)
                    n278 = call-poly <vilib>:"Delacor_lib_QMH_Enqueue Message (poly).vi"("error in"=w1153, "Message Data"=w1147, "Message"="Update state", "Message Queue in"=w1152) -> ("error out"=w1151:errorcluster)  [unwired: 6 in, 1 out]
                  }
                }
              }
            }
          }
          frame "Get current position" {
            # "Request to get current position (xxTP, {All})"
            n279 = Variant To Data(error in=w1176, type=T23 {"Module ID"=-1, "Address"=0, "Wait Notifier"=refnum, "wait for reply"=FALSE} ("Get current position Argument"), Variant=w1174) -> (data=w1172:T23, error out=w1175:errorcluster)
            n280 = Unbundle By Name(w1166) -> ("Instrument Channel"=w1165:string)
            n281 = Unbundle By Name(w1172) -> ("Address"=w1163:u8, "Module ID"=w1160:i32, "Wait Notifier"=w1171:refnum<notifier>, "wait for reply"=w1170:bool)
            n282 = Not Equal To 0?(x=w1163) -> (x != 0?=w1164:bool)
            n283 = case shown="True" w1164 {
              tunnel: w1163 -> [_ w1183]
              tunnel: w1165 -> [_ w1182]
              tunnel: [w1177 w1181] -> w1161
              tunnel: [_ w1180] -> w1162
              tunnel: w1160 -> [w1178 _]
              frame False {
                # "Address is 0. Broadcast not allowed for this command."
                n284 = call "Status Updated.vi"("Status"="Broadcast not allowed for this command. Use an address other than 0.", "Module ID"=w1178) -> ("error out"=w1177:errorcluster)  [unwired: 9 in]
              }
              frame True {
                w1186 = 0.0  # DBL
                # "Address not zero. Execute command."
                n285 = Format Into String(format string="%dTP\n", w1183) -> (resulting string=w1189:string)  [unwired: 2 in, 1 out]
                n286 = call "_QueryCommand.vi"("Command"=w1189, "Instrument Channel in"=w1182) -> ("error out"=w1181:errorcluster, "Response"=w1188:string)  [unwired: 7 in, 1 out]
                n287 = Match Pattern(string=w1188, regular expression="TP") -> (after substring=w1187:string)  [unwired: 1 in, 3 out]
                n288 = Decimal String To Number(string=w1187, default (0L)=w1186) -> (number=w1180:dbl)  [unwired: 1 in, 1 out]
              }
            }
            n289 = Bundle By Name(cluster=T41 {"Position"=0.0, "error"={"status"=FALSE, "code"=0, "source"=""}} ("Get current position (Reply Payload)"), "Position"=w1162, "error"=w1161) -> (w1169:T41)
            n290 = Merge Errors(w1175, w1161) -> (w1167:errorcluster)
            n291 = case shown="True" w1170 {
              tunnel: w1171 -> [_ w1191]
              tunnel: w1169 -> [_ w1190]
              frame False {
              }
              frame True {
                n292 = Send Notification(notification=w1190, notifier=w1191) -> ()  [unwired: 1 in, 2 out]
              }
            }
          }
          frame "Reset controller" {
            # "Request to power cycle the controller. Returns to Not referenced sate (xxRS, {All})"
            n293 = Variant To Data(error in=w1204, type=T24 {"Module ID"=-1, "Address"=0} ("Reset controller Argument"), Variant=w1203) -> (data=w1201:T24, error out=w1200:errorcluster)
            n294 = Unbundle By Name(w1195) -> ("Devices states"=w1193:T1[], "Instrument Channel"=w1198:string)
            n295 = Unbundle By Name(w1201) -> ("Address"=w1194:u8, "Module ID"=w1196:i32)
            n296 = Not Equal To 0?(x=w1194) -> (x != 0?=w1197:bool)
            n297 = case shown="True" w1197 {
              tunnel: w1200 -> [w1207 w1217]
              tunnel: [w1206 w1216] -> w1199
              tunnel: w1198 -> [_ w1214]
              tunnel: w1194 -> [_ w1211]
              tunnel: w1196 -> [w1208 _]
              tunnel: w1195 -> [w1205 w1213]
              tunnel: w1193 -> [_ _]
              tunnel: [w1205 w1212] -> w1192
              frame False {
                # "Address is 0. Broadcast not allowed for this command."
                n298 = call "Status Updated.vi"("error in (no error)"=w1207, "Status"="Broadcast not allowed for this command. Use an address other than 0.", "Module ID"=w1208) -> ("error out"=w1206:errorcluster)  [unwired: 8 in]
              }
              frame True {
                # "Address not zero. Execute command."
                n299 = Format Into String(format string="%dRS\n", w1211) -> (resulting string=w1215:string)  [unwired: 2 in, 1 out]
                n300 = for {
                  N: w1211 -> [_]
                  tunnel: [Device_state_--_enum."Not referenced" ("element")] -> w1210 mode=indexing
                }
                n301 = call "_SendCommand.vi"("error in"=w1217, "Command"=w1215, "Instrument Channel"=w1214) -> ("error out"=w1216:errorcluster)  [unwired: 7 in, 1 out]
                n302 = Bundle By Name(cluster=w1213, "Devices states"=w1210) -> (w1212:T6)
              }
            }
          }
          frame "---Exit and Error Handling---" {
            # "Separator - the following cases handle errors and exit messages."
          }
          frame "Error" {
            # "#CodeRecommended - If the module is running in standalone mode (External Launch = FALSE), this code will pop up an error dialog and call the 'Exit' message if an error occurs. Add more fine-grained error handling here."
            # "Error - Check the error message data and respond accordingly. This message is sent by the \"Error Handler\" VIs at the end of each loop in this application."
            n303 = property on="Property Node" class="Mod Admin"(reference=w1225) -> ("Accessors:External Launch"=w1224:bool, "Accessors:Module ID"=w1222:i32)  [unwired: 1 in, 2 out]
            n304 = Variant To Data(error in=w1232, type=errorcluster {"status"=FALSE, "code"=0, "source"=""} ("error constant"), Variant=w1226) -> (data=w1233:errorcluster, error out=w1230:errorcluster)
            n305 = call "Error Reported.vi"("Error"=w1233, "Module ID"=w1222) -> ()  [unwired: 9 in, 1 out]
            n306 = case shown="True" w1224 {
              tunnel: [w1238 _] -> w1229
              tunnel: w1223 -> [w1236 _]
              tunnel: w1233 -> [w1237 _]
              frame False {
                # "If the module is running standalone, then pop up an error dialog and call the \"Exit\" message."
                n307 = call <vilib>:"Simple Error Handler.vi"("error in (no error)"=w1237) -> ()  [unwired: 4 in, 5 out]
                n308 = call-poly <vilib>:"Delacor_lib_QMH_Enqueue Message (poly).vi"("Priority Message? (F)"=TRUE, "Message"="Exit", "Message Queue in"=w1236) -> ("error out"=w1238:errorcluster)  [unwired: 7 in, 1 out]
              }
              frame True {
                # "If the module was launched externally, calling the Error Reported broadcast VI is the only action performed by the \"Error\" message. The module's caller can then process the error appropriately."
              }
            }
            n309 = Merge Errors(w1230, w1229) -> (w1228:errorcluster)
            n310 = local write "error out"(w1228) -> ()
          }
          frame "Exit" {
            w1245 = 91  # 91: not all Exit messages will have an argument
            w1246 = TRUE  # Stop the VI
            # "Release the message queue reference"
            # "#CodeNeeded - Add any required cleanup code here."
            # "Exit - Exit the application."
            n311 = Variant To Data(error in=w1254, type=T9 {"Module ID"=-1, "Origin"="", "Exit via Stop Module Req?"=FALSE, "Wait for Module to stop?"=FALSE} ("Stop Argument"), Variant=w1244) -> (data=w1241:T9, error out=w1249:errorcluster)
            n312 = call <vilib>:"Clear Errors.vi"("error in (no error)"=w1249, "specific error code to clear (0: all)"=w1245) -> ("error out"=w1253:errorcluster)  [unwired: 4 in, 1 out]
            n313 = control-ref of="This VI"() -> (w1239:refnum<vi>)
            n314 = call-dynamic "Delacor_lib_QMH_Release Message Queue.vi"("error in"=w1253, "Message Queue"=w1248) -> ("error out"=w1252:errorcluster)  [unwired: 9 in]
            n315 = call "Handle Exit.vi"("Stop Argument"=w1241, "Module Admin in"=w1240, "VI reference"=w1239) -> ("error out"=w1250:errorcluster, "Wait for Stop?"=w1242:bool)  [unwired: 7 in]
            n316 = Merge Errors(w1252, w1250) -> (w1251:errorcluster)
          }
          frame Default {
            # "'Default' case only runs if there is a message that isn't defined in any of the other cases.  Output a programming error."
            n317 = property on="Property Node" class="Mod Admin"(reference=w1256) -> ("Accessors:Module ID"=w1255:i32)  [unwired: 1 in, 2 out]
            n318 = call "Module Name--constant.vi"("Module ID"=w1255) -> ("Module Name"=w1257:string)  [unwired: 10 in]
            n319 = xnode "Error Ring"("parameter 0"=w1258, "parameter 1"=w1257) -> ("error out"=w1262:errorcluster)
            n320 = Merge Errors(w1260, w1262) -> (w1261:errorcluster)
          }
          frame "Continuously check state" {
            # "Request to continuously monitor the device's marked by address until a given state has been achieved."
            n321 = Variant To Data(error in=w1287, type=T28 {"Module ID"=-1, "Address"=0, "Desired state"=enum."Configuration", "Timeout"=0} ("Continuously check state Argument"), Variant=w1286) -> (data=w1284:T28, error out=w1283:errorcluster)
            n322 = Unbundle By Name(w1281) -> ("Instrument Channel"=w1275:string, "Devices states"=w1274:T1[])
            n323 = Unbundle By Name(w1284) -> ("Timeout"=w1278:i32, "Module ID"=w1276:i32, "Address"=w1273:u8, "Desired state"=w1271:T1)
            n324 = Index Array(array=w1274, index=w1273) -> (element=w1272:T1)
            n325 = Bundle By Name(cluster=T42 {"Timeout"=0, "Instrument Channel"="", "Address"=0, "Current state"=enum."Configuration", "Desired state"=enum."Configuration", "Module ID"=0} ("event data"), "Instrument Channel"=w1275, "Current state"=w1272, "Timeout"=w1278, "Module ID"=w1276, "Address"=w1273, "Desired state"=w1271) -> (w1277:T42)
            n326 = call "Wake HL.vi"("error in (no error)"=w1283, "event data"=w1277, "event cluster"=w1280) -> ("error out"=w1282:errorcluster)  [unwired: 8 in]
          }
          frame "Stop checking state" {
            # "Request to stop continuous monitoring of the device state marked by address."
            n327 = Variant To Data(error in=w1296, type=T29 {"Module ID"=-1, "Address"=0} ("Stop checking state Argument"), Variant=w1294) -> (data=w1292:T29, error out=w1291:errorcluster)
            n328 = Unbundle By Name(w1292) -> ("Address"=w1288:u8)  [unwired: 1 out]
            n329 = call "Sleep HL.vi"("error in (no error)"=w1291, "event data"=w1288, "event cluster"=w1289) -> ("error out"=w1290:errorcluster)  [unwired: 8 in]
          }
          frame "Configure simultaneous move" {
            # "Request to configure simultaneous started move. If xxSEnn sent, it configures the target position for the device with address xx, if address is 0, all devices will be configured with the same target position {Ready}."
            n330 = Unbundle By Name(w1303) -> ("Instrument Channel"=w1302:string, "Devices states"=w1300:T1[])
            n331 = Variant To Data(error in=w1310, type=T30 {"Module ID"=-1, "Address"=0, "Position"=0.0} ("Configure simultaneous move Argument"), Variant=w1309) -> (data=w1307:T30, error out=w1306:errorcluster)
            n332 = Unbundle By Name(w1307) -> ("Module ID"=w1297:i32, "Address"=w1299:u8, "Position"=w1304:dbl)
            n333 = Decrement(x=w1299) -> (x-1=w1298:u8)
            n334 = Index Array(array=w1300, index=w1298) -> (element=w1301:T1)
            n335 = case shown="\"Ready\"" w1301 {
              selector: w1301 -> [w1315 _]
              tunnel: w1306 -> [w1318 w1326]
              tunnel: [w1317 w1319] -> w1305
              tunnel: w1302 -> [_ w1325]
              tunnel: w1304 -> [_ w1324]
              tunnel: w1299 -> [_ w1323]
              tunnel: w1297 -> [w1311 w1321]
              frame Default {
                n336 = property on="Device state" class="Enum (strict)"() -> ("Strings []"=w1316:string[])  [unwired: 2 in, 2 out]
                n337 = Index Array(array=w1316, index=w1315) -> (element=w1313:string)
                n338 = Format Into String(format string="Simultaneous movement only allowed in Ready state. Current state: %s." ("Status"), w1313) -> (resulting string=w1312:string)  [unwired: 2 in, 1 out]
                n339 = call "Status Updated.vi"("error in (no error)"=w1318, "Status"=w1312, "Module ID"=w1311) -> ("error out"=w1317:errorcluster)  [unwired: 8 in]
              }
              frame "Ready" {
                n340 = Format Into String(format string="%dSE%0.3f\n", w1323, w1324) -> (resulting string=w1328:string)  [unwired: 2 in, 1 out]
                n341 = call "_SendCommand.vi"("error in"=w1326, "Command"=w1328, "Instrument Channel"=w1325) -> ("error out"=w1322:errorcluster)  [unwired: 7 in, 1 out]
                n342 = call "Status Updated.vi"("error in (no error)"=w1322, "Status"="Simultaneous movement configured.", "Module ID"=w1321) -> ("error out"=w1319:errorcluster)  [unwired: 8 in]
              }
            }
          }
          frame "Get simultaneous move config" {
            # "Request to get configuration of the device idenfied by address, xxSE? {Ready}."
            n343 = Unbundle By Name(w1338) -> ("Instrument Channel"=w1337:string, "Devices states"=w1336:T1[])
            n344 = Variant To Data(error in=w1348, type=T31 {"Module ID"=-1, "Address"=0, "Wait Notifier"=refnum, "wait for reply"=FALSE} ("Get simultaneous move config Argument"), Variant=w1346) -> (data=w1344:T31, error out=w1347:errorcluster)
            n345 = Unbundle By Name(w1344) -> ("Address"=w1332:u8, "Module ID"=w1331:i32, "Wait Notifier"=w1343:refnum<notifier>, "wait for reply"=w1342:bool)
            n346 = Decrement(x=w1332) -> (x-1=w1334:u8)
            n347 = Not Equal To 0?(x=w1332) -> (x != 0?=w1333:bool)
            n348 = Index Array(array=w1336, index=w1334) -> (element=w1335:T1)
            n349 = case shown="True" w1333 {
              tunnel: [w1350 w1357] -> w1329
              tunnel: w1335 -> [_ w1356]
              tunnel: w1337 -> [_ w1355]
              tunnel: w1332 -> [_ w1354]
              tunnel: w1331 -> [w1349 w1353]
              tunnel: [_ w1352] -> w1330
              frame False {
                # "Address is 0. Broadcast not allowed."
                n350 = call "Status Updated.vi"("Status"="Broadcast not allowed for this command. Use an address other than 0.", "Module ID"=w1349) -> ("error out"=w1350:errorcluster)  [unwired: 9 in]
              }
              frame True {
                # "Address not zero. Execute command."
                n351 = case shown="\"Ready\"" w1356 {
                  selector: w1356 -> [w1361 _]
                  tunnel: [w1364 w1368] -> w1357
                  tunnel: w1355 -> [_ w1367]
                  tunnel: w1354 -> [_ w1369]
                  tunnel: w1353 -> [w1363 _]
                  tunnel: [_ w1365] -> w1352
                  frame Default {
                    n352 = property on="Device state" class="Enum (strict)"() -> ("Strings []"=w1362:string[])  [unwired: 2 in, 2 out]
                    n353 = Index Array(array=w1362, index=w1361) -> (element=w1359:string)
                    n354 = Format Into String(format string="Command only allowed in Ready state. Current state: %s." ("Status"), w1359) -> (resulting string=w1358:string)  [unwired: 2 in, 1 out]
                    n355 = call "Status Updated.vi"("Status"=w1358, "Module ID"=w1363) -> ("error out"=w1364:errorcluster)  [unwired: 9 in]
                  }
                  frame "Ready" {
                    n356 = Format Into String(format string="%dSE?\n", w1369) -> (resulting string=w1366:string)  [unwired: 2 in, 1 out]
                    n357 = call "_QueryCommand.vi"("Command"=w1366, "Instrument Channel in"=w1367) -> ("error out"=w1368:errorcluster, "Response"=w1365:string)  [unwired: 7 in, 1 out]
                  }
                }
              }
            }
            n358 = Bundle By Name(cluster=T43 {"Response"="", "error"={"status"=FALSE, "code"=0, "source"=""}} ("Get simultaneous move config (Reply Payload)"), "Response"=w1330, "error"=w1329) -> (w1341:T43)
            n359 = Merge Errors(w1347, w1329) -> (w1339:errorcluster)
            n360 = case shown="True" w1342 {
              tunnel: w1343 -> [_ w1372]
              tunnel: w1341 -> [_ w1371]
              frame False {
              }
              frame True {
                n361 = Send Notification(notification=w1371, notifier=w1372) -> ()  [unwired: 1 in, 2 out]
              }
            }
          }
          frame "Execute simultaneous move" {
            # "Request to execute simultaneous move. Configure simultaneous move beforewards."
            n362 = Variant To Data(error in=w1385, type=T32 {"Module ID"=-1, "Boolean"=FALSE} ("Execute simultaneous move Argument"), Variant=w1384) -> (data=w1382:T32, error out=w1381:errorcluster)
            n363 = Unbundle By Name(w1379) -> ("Instrument Channel"=w1378:string, "Devices states"=w1376:T1[])
            n364 = Unbundle By Name(w1382) -> ("Module ID"=w1377:i32)
            n365 = Equal?(x=w1376, y=Device_state_--_enum."Ready" ("Device state")) -> (x = y?=w1374:bool[])
            n366 = And Array Elements(Boolean array=w1374) -> (logical AND=w1373:bool)
            n367 = case shown="True" w1373 {
              tunnel: [w1389 w1393] -> w1380
              tunnel: w1378 -> [_ w1391]
              tunnel: w1377 -> [w1388 _]
              tunnel: w1381 -> [w1386 w1392]
              frame False {
                n368 = call "Status Updated.vi"("error in (no error)"=w1386, "Status"="Command only allowed if all FCRs are in  Ready state.", "Module ID"=w1388) -> ("error out"=w1389:errorcluster)  [unwired: 8 in]
              }
              frame True {
                n369 = call "_SendCommand.vi"("error in"=w1392, "Command"="ES\n" ("format string"), "Instrument Channel"=w1391) -> ("error out"=w1393:errorcluster)  [unwired: 7 in, 1 out]
              }
            }
          }
        }
        n370 = call-dynamic "Delacor_lib_QMH_Error Handler - Message Handling Loop.vi"("error in"=w480, "Message Queue in"=w470) -> ("dup error in"=w477:errorcluster)  [unwired: 8 in, 1 out]
      }
      n371 = while {
        tunnel: w31 -> [w90]
        shift-right: [w93] -> w39
        shift-left: w37 -> [w94]
        tunnel: [w95] -> w41
        tunnel: w36 -> [w91]
        stop <- w92 stop-if-true
        # "Event Handling Loop"
        n372 = event "DQMH_EVENT_MAIN" shown="[28] <FCR100 Request Events.Execute simultaneous move>: User Event" {
          selector: w94 -> [_ _ _ _ _ _ _ _ _ _ _ _ _ _ _ _ _ _ _ _ _ _ _ _ _ _ _ _ _]
          dyn-events: [_ _ _ _ _ _ _ _ _ _ _ _ _ _ _ _ _ _ _ _ _ _ _ _ _ _ _ _ _] -> w93
          timeout: _ -> [_ _ _ _ _ _ _ _ _ _ _ _ _ _ _ _ _ _ _ _ _ _ _ _ _ _ _ _ _]
          tunnel: [_ _ _ _ w137 _ _ _ _ _ _ _ _ _ _ _ _ _ _ _ _ _ _ _ _ _ _ _ _] -> w92
          tunnel: w90 -> [_ _ _ _ w140 w164 w177 w190 w202 w214 w228 w241 w255 w268 w282 w297 w310 w323 w337 w343 w359 w372 w385 w397 w411 w423 w436 w450 w462]
          tunnel: [_ _ w114 _ w141 w155 w170 w183 w195 w207 w219 w233 w246 w260 w274 w287 w302 w315 w328 w346 w352 w366 w378 w390 w403 w416 w428 w441 w455] -> w96
          tunnel: w91 -> [w97 w104 w112 w118 w139 w162 w175 w188 w200 w212 w226 w239 w253 w266 w280 w295 w308 w321 w335 w344 w357 w370 w383 w395 w409 w421 w434 w448 w460]
          event User Event {
            # "Another Module called the \"Show Panel\" API Method."
            n373 = event-data() -> ("Module ID"=w98:i32)  [unwired: 1 in]
            n374 = call "Addressed to This Module.vi"("Module ID from Argument"=w98, "Module Admin"=w97) -> ("Addressed to this instance?"=w99:bool)  [unwired: 8 in, 1 out]
            n375 = case shown="True" w99 {
              tunnel: w97 -> [_ w101]
              frame False {
              }
              frame True {
                # "Show the panel of this VI, and send a status updated message to let listeners know."
                n376 = property on="Property Node" class="Mod Admin"(reference=w101) -> ("Accessors:Module ID"=w100:i32)  [unwired: 1 in, 2 out]
                n377 = control-ref of="This VI"() -> (w103:refnum<vi>)
                n378 = call "Open VI Panel.vi"("VI"=w103) -> ()  [unwired: 10 in, 1 out]
                n379 = call "Status Updated.vi"("Status"="Panel shown." ("format string"), "Module ID"=w100) -> ()  [unwired: 9 in, 1 out]
              }
            }
          }
          event User Event {
            # "Another Module called the \"Hide Panel\" API Method."
            n380 = event-data() -> ("Module ID"=w105:i32)  [unwired: 1 in]
            n381 = call "Addressed to This Module.vi"("Module ID from Argument"=w105, "Module Admin"=w104) -> ("Addressed to this instance?"=w106:bool)  [unwired: 8 in, 1 out]
            n382 = case shown="True" w106 {
              tunnel: w104 -> [_ w108]
              frame False {
              }
              frame True {
                # "Hide the panel of this VI, and send a status updated message to let listeners know."
                n383 = property on="Property Node" class="Mod Admin"(reference=w108) -> ("Accessors:Module ID"=w107:i32)  [unwired: 1 in, 2 out]
                n384 = control-ref of="This VI"() -> (w110:refnum<vi>)
                n385 = call "Hide VI Panel.vi"("VI"=w110) -> ()  [unwired: 10 in, 1 out]
                n386 = call "Status Updated.vi"("Status"="Panel hidden." ("format string"), "Module ID"=w107) -> ()  [unwired: 9 in, 1 out]
              }
            }
          }
          event User Event {
            # "For cloneable running as singleton, broadcast that the module is running."
            n387 = event-data() -> ("Module ID"=w111:i32)  [unwired: 1 in]
            n388 = call "Addressed to This Module.vi"("Module ID from Argument"=w111, "Module Admin"=w112) -> ("Addressed to this instance?"=w113:bool)  [unwired: 8 in, 1 out]
            n389 = case shown="True" w113 {
              tunnel: [_ w117] -> w114
              tunnel: w111 -> [_ w116]
              frame False {
              }
              frame True {
                n390 = call "Update Module Execution Status.vi"("Running?"=TRUE, "Module ID"=w116) -> ("error out"=w117:errorcluster)  [unwired: 9 in]
              }
            }
          }
          event User Event {
            # "Another Module called the \"Show Diagram\" API Method. This event is used for debugging."
            n391 = event-data() -> ("Module ID"=w119:i32)  [unwired: 1 in]
            n392 = call "Addressed to This Module.vi"("Module ID from Argument"=w119, "Module Admin"=w118) -> ("Addressed to this instance?"=w120:bool)  [unwired: 8 in, 1 out]
            n393 = case shown="True" w120 {
              tunnel: w118 -> [_ w121]
              frame False {
              }
              frame True {
                n394 = disable-structure shown="RUN_TIME_ENGINE==False" {
                  disable-tunnel: w121 -> [w122 _]
                  frame condition #0 (active) {
                    # "functionality not available in exe"
                    n395 = invoke on="Invoke Node" class="VI" method="Lock State.Get"() -> (error out=w128:errorcluster, "Get Lock State"=w127:T8, "pwd in cache"=w124:bool)  [unwired: 4 in, 1 out]
                    n396 = Equal?(x=T8."Password-protected", y=w127) -> (x = y?=w125:bool)
                    n397 = Compound Arithmetic op=AND(w125, invert w124) -> (w123:bool)
                    n398 = case shown="False" w123 {
                      tunnel: w128 -> [w133 _]
                      tunnel: w122 -> [w130 _]
                      frame False {
                        n399 = property on="Property Node" class="Mod Admin"(reference=w130) -> ("Accessors:Module ID"=w129:i32)  [unwired: 1 in, 2 out]
                        n400 = property on="Property Node" class="VI"(error in=w133, "BDWin.Open"=TRUE ("Block Diagram Window:Open")) -> ()  [unwired: 1 in, 2 out]
                        n401 = call "Status Updated.vi"("Status"="Block Diagram shown." ("format string"), "Module ID"=w129) -> ()  [unwired: 9 in, 1 out]
                      }
                      frame True {
                        # "Password-protected VI, and the password is not in the cache. Do not show the diagram."
                      }
                    }
                  }
                  frame condition #1 {
                  }
                }
              }
            }
          }
          event User Event {
            # "Another Module called the \"Stop Module\" API Method  or the Message Handling Loop below."
            n402 = event-data() -> ("Module ID"=w135:i32, "Wait for Module to stop?"=w136:bool, "Origin"=w134:string)  [unwired: 1 in]
            n403 = call "Addressed to This Module.vi"("Module ID from Argument"=w135, "Module Admin"=w139) -> ("Addressed to this instance?"=w138:bool)  [unwired: 8 in, 1 out]
            n404 = case shown="True" w138 {
              tunnel: [_ w153] -> w141
              tunnel: w140 -> [_ w149]
              tunnel: [_ TRUE] -> w137
              tunnel: w136 -> [_ w144]
              tunnel: w135 -> [_ w146]
              tunnel: w134 -> [_ w142]
              frame False {
              }
              frame True {
                # "The event can get fired from the Exit message. The queue gets destroyed there. In this case, the Enqueue VI will return error 1. It is safe to ignore, because the module is already exiting."
                n405 = local write "Status"(w142) -> ()
                n406 = Bundle By Name(cluster=T9 {"Module ID"=-1, "Origin"="", "Exit via Stop Module Req?"=FALSE, "Wait for Module to stop?"=FALSE} ("Stop Argument"), "Module ID"=w146, "Exit via Stop Module Req?"=TRUE, "Wait for Module to stop?"=w144) -> (w143:T9)
                n407 = call-poly <vilib>:"Delacor_lib_QMH_Enqueue Message (poly).vi"("Priority Message? (F)"=TRUE, "Message Data"=w143, "Message"="Exit", "Message Queue in"=w149) -> ("error out"=w154:errorcluster)  [unwired: 6 in, 1 out]
                n408 = call <vilib>:"Clear Errors.vi"("error in (no error)"=w154, "specific error code to clear (0: all)"=1) -> ("error out"=w153:errorcluster)  [unwired: 4 in, 1 out]
              }
            }
          }
          event User Event {
            # "Another Module called the \"Connect with dialog\" API Method."
            n409 = event-data() -> ("Module ID"=w159:i32, "Baud Rate"=w158:u32, "Wait Notifier"=w157:refnum<notifier>, "wait for reply"=w156:bool)  [unwired: 1 in]
            n410 = Bundle(cluster=T10 {"Module ID"=-1, "Baud Rate"=115200, "Wait Notifier"=refnum, "wait for reply"=FALSE} ("Connect with dialog Argument"), "Module ID"=w159, "Baud Rate"=w158, "Wait Notifier"=w157, "wait for reply"=w156) -> (w160:T10)
            n411 = call "Addressed to This Module.vi"("Module ID from Argument"=w159, "Module Admin"=w162) -> ("Addressed to this instance?"=w163:bool)  [unwired: 8 in, 1 out]
            n412 = case shown="True" w163 {
              tunnel: w164 -> [_ w168]
              tunnel: w160 -> [_ w166]
              tunnel: [_ w165] -> w155
              frame False {
              }
              frame True {
                n413 = call-poly <vilib>:"Delacor_lib_QMH_Enqueue Message (poly).vi"("Message Data"=w166, "Message"="Connect with dialog", "Message Queue in"=w168) -> ("error out"=w165:errorcluster)  [unwired: 7 in, 1 out]
              }
            }
          }
          event User Event {
            # "Another Module called the \"Change configuration state\" API Method."
            n414 = event-data() -> ("Module ID"=w172:i32, "Enter/(leave)"=w171:bool, "Address"=w169:u8)  [unwired: 1 in]
            n415 = Bundle(cluster=T11 {"Module ID"=-1, "Enter/(leave)"=FALSE, "Address"=0} ("Change configuration state Argument"), "Module ID"=w172, "Enter/(leave)"=w171, "Address"=w169) -> (w173:T11)
            n416 = call "Addressed to This Module.vi"("Module ID from Argument"=w172, "Module Admin"=w175) -> ("Addressed to this instance?"=w176:bool)  [unwired: 8 in, 1 out]
            n417 = case shown="True" w176 {
              tunnel: w177 -> [_ w181]
              tunnel: w173 -> [_ w179]
              tunnel: [_ w178] -> w170
              frame False {
              }
              frame True {
                n418 = call-poly <vilib>:"Delacor_lib_QMH_Enqueue Message (poly).vi"("Message Data"=w179, "Message"="Change configuration state", "Message Queue in"=w181) -> ("error out"=w178:errorcluster)  [unwired: 7 in, 1 out]
              }
            }
          }
          event User Event {
            # "Another Module called the \"Change disable state\" API Method."
            n419 = event-data() -> ("Module ID"=w185:i32, "Enter/Leave"=w184:bool, "Address"=w182:u8)  [unwired: 1 in]
            n420 = Bundle(cluster=T12 {"Module ID"=-1, "Enter/Leave"=FALSE, "Address"=0} ("Change disable state Argument"), "Module ID"=w185, "Enter/Leave"=w184, "Address"=w182) -> (w186:T12)
            n421 = call "Addressed to This Module.vi"("Module ID from Argument"=w185, "Module Admin"=w188) -> ("Addressed to this instance?"=w189:bool)  [unwired: 8 in, 1 out]
            n422 = case shown="True" w189 {
              tunnel: w190 -> [_ w194]
              tunnel: w186 -> [_ w192]
              tunnel: [_ w191] -> w183
              frame False {
              }
              frame True {
                n423 = call-poly <vilib>:"Delacor_lib_QMH_Enqueue Message (poly).vi"("Message Data"=w192, "Message"="Change disable state", "Message Queue in"=w194) -> ("error out"=w191:errorcluster)  [unwired: 7 in, 1 out]
              }
            }
          }
          event User Event {
            # "Another Module called the \"Search Home\" API Method."
            n424 = event-data() -> ("Module ID"=w197:i32, "Address"=w196:u8)  [unwired: 1 in]
            n425 = Bundle(cluster=T13 {"Module ID"=-1, "Address"=0} ("Search Home Argument"), "Module ID"=w197, "Address"=w196) -> (w198:T13)
            n426 = call "Addressed to This Module.vi"("Module ID from Argument"=w197, "Module Admin"=w200) -> ("Addressed to this instance?"=w201:bool)  [unwired: 8 in, 1 out]
            n427 = case shown="True" w201 {
              tunnel: w202 -> [_ w206]
              tunnel: w198 -> [_ w204]
              tunnel: [_ w203] -> w195
              frame False {
              }
              frame True {
                n428 = call-poly <vilib>:"Delacor_lib_QMH_Enqueue Message (poly).vi"("Message Data"=w204, "Message"="Search Home", "Message Queue in"=w206) -> ("error out"=w203:errorcluster)  [unwired: 7 in, 1 out]
              }
            }
          }
          event User Event {
            # "Another Module called the \"Stop movement\" API Method."
            n429 = event-data() -> ("Module ID"=w209:i32, "Address"=w208:u8)  [unwired: 1 in]
            n430 = Bundle(cluster=T14 {"Module ID"=-1, "Address"=0} ("Stop movement Argument"), "Module ID"=w209, "Address"=w208) -> (w210:T14)
            n431 = call "Addressed to This Module.vi"("Module ID from Argument"=w209, "Module Admin"=w212) -> ("Addressed to this instance?"=w213:bool)  [unwired: 8 in, 1 out]
            n432 = case shown="True" w213 {
              tunnel: w214 -> [_ w218]
              tunnel: w210 -> [_ w216]
              tunnel: [_ w215] -> w207
              frame False {
              }
              frame True {
                n433 = call-poly <vilib>:"Delacor_lib_QMH_Enqueue Message (poly).vi"("Message Data"=w216, "Message"="Stop movement", "Message Queue in"=w218) -> ("error out"=w215:errorcluster)  [unwired: 7 in, 1 out]
              }
            }
          }
          event User Event {
            # "Another Module called the \"Get state\" API Method."
            n434 = event-data() -> ("Module ID"=w223:i32, "Address"=w222:u8, "Wait Notifier"=w221:refnum<notifier>, "wait for reply"=w220:bool)  [unwired: 1 in]
            n435 = Bundle(cluster=T15 {"Module ID"=-1, "Address"=0, "Wait Notifier"=refnum, "wait for reply"=FALSE} ("Get state Argument"), "Module ID"=w223, "Address"=w222, "Wait Notifier"=w221, "wait for reply"=w220) -> (w224:T15)
            n436 = call "Addressed to This Module.vi"("Module ID from Argument"=w223, "Module Admin"=w226) -> ("Addressed to this instance?"=w227:bool)  [unwired: 8 in, 1 out]
            n437 = case shown="True" w227 {
              tunnel: w228 -> [_ w232]
              tunnel: w224 -> [_ w230]
              tunnel: [_ w229] -> w219
              frame False {
              }
              frame True {
                n438 = call-poly <vilib>:"Delacor_lib_QMH_Enqueue Message (poly).vi"("Message Data"=w230, "Message"="Get state", "Message Queue in"=w232) -> ("error out"=w229:errorcluster)  [unwired: 7 in, 1 out]
              }
            }
          }
          event User Event {
            # "Another Module called the \"Set acceleration\" API Method."
            n439 = event-data() -> ("Module ID"=w236:i32, "Address"=w235:u8, "Acceleration"=w234:u16)  [unwired: 1 in]
            n440 = Bundle(cluster=T16 {"Module ID"=-1, "Address"=0, "Acceleration"=0} ("Set acceleration Argument"), "Module ID"=w236, "Address"=w235, "Acceleration"=w234) -> (w237:T16)
            n441 = call "Addressed to This Module.vi"("Module ID from Argument"=w236, "Module Admin"=w239) -> ("Addressed to this instance?"=w240:bool)  [unwired: 8 in, 1 out]
            n442 = case shown="True" w240 {
              tunnel: w241 -> [_ w245]
              tunnel: w237 -> [_ w243]
              tunnel: [_ w242] -> w233
              frame False {
              }
              frame True {
                n443 = call-poly <vilib>:"Delacor_lib_QMH_Enqueue Message (poly).vi"("Message Data"=w243, "Message"="Set acceleration", "Message Queue in"=w245) -> ("error out"=w242:errorcluster)  [unwired: 7 in, 1 out]
              }
            }
          }
          event User Event {
            # "Another Module called the \"Get acceleration\" API Method."
            n444 = event-data() -> ("Module ID"=w250:i32, "Address"=w249:u8, "Wait Notifier"=w248:refnum<notifier>, "wait for reply"=w247:bool)  [unwired: 1 in]
            n445 = Bundle(cluster=T17 {"Module ID"=-1, "Address"=0, "Wait Notifier"=refnum, "wait for reply"=FALSE} ("Get acceleration Argument"), "Module ID"=w250, "Address"=w249, "Wait Notifier"=w248, "wait for reply"=w247) -> (w251:T17)
            n446 = call "Addressed to This Module.vi"("Module ID from Argument"=w250, "Module Admin"=w253) -> ("Addressed to this instance?"=w254:bool)  [unwired: 8 in, 1 out]
            n447 = case shown="True" w254 {
              tunnel: w255 -> [_ w259]
              tunnel: w251 -> [_ w257]
              tunnel: [_ w256] -> w246
              frame False {
              }
              frame True {
                n448 = call-poly <vilib>:"Delacor_lib_QMH_Enqueue Message (poly).vi"("Message Data"=w257, "Message"="Get acceleration", "Message Queue in"=w259) -> ("error out"=w256:errorcluster)  [unwired: 7 in, 1 out]
              }
            }
          }
          event User Event {
            # "Another Module called the \"Set velocity\" API Method."
            n449 = event-data() -> ("Module ID"=w263:i32, "Address"=w262:u8, "Velocity"=w261:u16)  [unwired: 1 in]
            n450 = Bundle(cluster=T18 {"Module ID"=-1, "Address"=0, "Velocity"=0} ("Set velocity Argument"), "Module ID"=w263, "Address"=w262, "Velocity"=w261) -> (w264:T18)
            n451 = call "Addressed to This Module.vi"("Module ID from Argument"=w263, "Module Admin"=w266) -> ("Addressed to this instance?"=w267:bool)  [unwired: 8 in, 1 out]
            n452 = case shown="True" w267 {
              tunnel: w268 -> [_ w272]
              tunnel: w264 -> [_ w270]
              tunnel: [_ w269] -> w260
              frame False {
              }
              frame True {
                n453 = call-poly <vilib>:"Delacor_lib_QMH_Enqueue Message (poly).vi"("Message Data"=w270, "Message"="Set velocity", "Message Queue in"=w272) -> ("error out"=w269:errorcluster)  [unwired: 7 in, 1 out]
              }
            }
          }
          event User Event {
            # "Another Module called the \"Get velocity\" API Method."
            n454 = event-data() -> ("Module ID"=w273:i32, "Address"=w277:u8, "Wait Notifier"=w276:refnum<notifier>, "wait for reply"=w275:bool)  [unwired: 1 in]
            n455 = Bundle(cluster=T19 {"Module ID"=-1, "Address"=0, "Wait Notifier"=refnum, "wait for reply"=FALSE} ("Get velocity Argument"), "Module ID"=w273, "Address"=w277, "Wait Notifier"=w276, "wait for reply"=w275) -> (w278:T19)
            n456 = call "Addressed to This Module.vi"("Module ID from Argument"=w273, "Module Admin"=w280) -> ("Addressed to this instance?"=w281:bool)  [unwired: 8 in, 1 out]
            n457 = case shown="True" w281 {
              tunnel: w282 -> [_ w286]
              tunnel: w278 -> [_ w284]
              tunnel: [_ w283] -> w274
              frame False {
              }
              frame True {
                n458 = call-poly <vilib>:"Delacor_lib_QMH_Enqueue Message (poly).vi"("Message Data"=w284, "Message"="Get velocity", "Message Queue in"=w286) -> ("error out"=w283:errorcluster)  [unwired: 7 in, 1 out]
              }
            }
          }
          event User Event {
            # "Another Module called the \"Get ETA\" API Method."
            n459 = event-data() -> ("Module ID"=w292:i32, "Address"=w291:u8, "Position"=w290:dbl, "Wait Notifier"=w289:refnum<notifier>, "wait for reply"=w288:bool)  [unwired: 1 in]
            n460 = Bundle(cluster=T20 {"Module ID"=-1, "Address"=0, "Position"=0.0, "Wait Notifier"=refnum, "wait for reply"=FALSE} ("Get ETA Argument"), "Module ID"=w292, "Address"=w291, "Position"=w290, "Wait Notifier"=w289, "wait for reply"=w288) -> (w293:T20)
            n461 = call "Addressed to This Module.vi"("Module ID from Argument"=w292, "Module Admin"=w295) -> ("Addressed to this instance?"=w296:bool)  [unwired: 8 in, 1 out]
            n462 = case shown="True" w296 {
              tunnel: w297 -> [_ w301]
              tunnel: w293 -> [_ w299]
              tunnel: [_ w298] -> w287
              frame False {
              }
              frame True {
                n463 = call-poly <vilib>:"Delacor_lib_QMH_Enqueue Message (poly).vi"("Message Data"=w299, "Message"="Get ETA", "Message Queue in"=w301) -> ("error out"=w298:errorcluster)  [unwired: 7 in, 1 out]
              }
            }
          }
          event User Event {
            # "Another Module called the \"Move absolute\" API Method."
            n464 = event-data() -> ("Module ID"=w305:i32, "Address"=w304:u8, "Position"=w303:dbl)  [unwired: 1 in]
            n465 = Bundle(cluster=T21 {"Module ID"=-1, "Address"=0, "Position"=0.0} ("Move absolute Argument"), "Module ID"=w305, "Address"=w304, "Position"=w303) -> (w306:T21)
            n466 = call "Addressed to This Module.vi"("Module ID from Argument"=w305, "Module Admin"=w308) -> ("Addressed to this instance?"=w309:bool)  [unwired: 8 in, 1 out]
            n467 = case shown="True" w309 {
              tunnel: w310 -> [_ w314]
              tunnel: w306 -> [_ w312]
              tunnel: [_ w311] -> w302
              frame False {
              }
              frame True {
                n468 = call-poly <vilib>:"Delacor_lib_QMH_Enqueue Message (poly).vi"("Message Data"=w312, "Message"="Move absolute", "Message Queue in"=w314) -> ("error out"=w311:errorcluster)  [unwired: 7 in, 1 out]
              }
            }
          }
          event User Event {
            # "Another Module called the \"Move relative\" API Method."
            n469 = event-data() -> ("Module ID"=w318:i32, "Address"=w317:u8, "Position"=w316:dbl)  [unwired: 1 in]
            n470 = Bundle(cluster=T22 {"Module ID"=-1, "Address"=0, "Position"=0.0} ("Move relative Argument"), "Module ID"=w318, "Address"=w317, "Position"=w316) -> (w319:T22)
            n471 = call "Addressed to This Module.vi"("Module ID from Argument"=w318, "Module Admin"=w321) -> ("Addressed to this instance?"=w322:bool)  [unwired: 8 in, 1 out]
            n472 = case shown="True" w322 {
              tunnel: w323 -> [_ w327]
              tunnel: w319 -> [_ w325]
              tunnel: [_ w324] -> w315
              frame False {
              }
              frame True {
                n473 = call-poly <vilib>:"Delacor_lib_QMH_Enqueue Message (poly).vi"("Message Data"=w325, "Message"="Move relative", "Message Queue in"=w327) -> ("error out"=w324:errorcluster)  [unwired: 7 in, 1 out]
              }
            }
          }
          event User Event {
            # "Another Module called the \"Get current position\" API Method."
            n474 = event-data() -> ("Module ID"=w332:i32, "Address"=w331:u8, "Wait Notifier"=w330:refnum<notifier>, "wait for reply"=w329:bool)  [unwired: 1 in]
            n475 = Bundle(cluster=T23 {"Module ID"=-1, "Address"=0, "Wait Notifier"=refnum, "wait for reply"=FALSE} ("Get current position Argument"), "Module ID"=w332, "Address"=w331, "Wait Notifier"=w330, "wait for reply"=w329) -> (w333:T23)
            n476 = call "Addressed to This Module.vi"("Module ID from Argument"=w332, "Module Admin"=w335) -> ("Addressed to this instance?"=w336:bool)  [unwired: 8 in, 1 out]
            n477 = case shown="True" w336 {
              tunnel: w337 -> [_ w341]
              tunnel: w333 -> [_ w339]
              tunnel: [_ w338] -> w328
              frame False {
              }
              frame True {
                n478 = call-poly <vilib>:"Delacor_lib_QMH_Enqueue Message (poly).vi"("Message Data"=w339, "Message"="Get current position", "Message Queue in"=w341) -> ("error out"=w338:errorcluster)  [unwired: 7 in, 1 out]
              }
            }
          }
          event Panel Close? {
            w345 = TRUE  # Discard the event, the MHL is responsible for closing and stopping this VI.
            # "Hide the panel or send the 'Exit' message if the user clicks the 'X' on the module main VI panel."
            n479 = event-data() -> ()  [unwired: 1 in, 1 out]
            n480 = property on="Property Node" class="Mod Admin"(reference=w344) -> ("Accessors:External Launch"=w342:bool)  [unwired: 1 in, 2 out]
            n481 = case shown="True" w342 {
              tunnel: w343 -> [_ w350]
              tunnel: [_ w351] -> w346
              frame True {
                # "If externally launched, clicking the 'X' hides the panel, but doesn't close it."
                n482 = control-ref of="This VI"() -> (w347:refnum<vi>)
                n483 = call "Hide VI Panel.vi"("VI"=w347) -> ()  [unwired: 10 in, 1 out]
              }
              frame False {
                # "If run as a stand-alone VI, clicking the panel 'X' stops the VI."
                n484 = call-poly <vilib>:"Delacor_lib_QMH_Enqueue Message (poly).vi"("Priority Message? (F)"=TRUE, "Message"="Exit", "Message Queue in"=w350) -> ("error out"=w351:errorcluster)  [unwired: 7 in, 1 out]
              }
            }
            n485 = event-data ("Event Filter Node")("Discard?"=w345) -> ()  [unwired: 1 in, 1 out]
          }
          event User Event {
            # "Another Module called the \"Reset controller\" API Method."
            n486 = event-data() -> ("Module ID"=w354:i32, "Address"=w353:u8)  [unwired: 1 in]
            n487 = Bundle(cluster=T24 {"Module ID"=-1, "Address"=0} ("Reset controller Argument"), "Module ID"=w354, "Address"=w353) -> (w355:T24)
            n488 = call "Addressed to This Module.vi"("Module ID from Argument"=w354, "Module Admin"=w357) -> ("Addressed to this instance?"=w358:bool)  [unwired: 8 in, 1 out]
            n489 = case shown="True" w358 {
              tunnel: w359 -> [_ w363]
              tunnel: w355 -> [_ w361]
              tunnel: [_ w360] -> w352
              frame False {
              }
              frame True {
                n490 = call-poly <vilib>:"Delacor_lib_QMH_Enqueue Message (poly).vi"("Message Data"=w361, "Message"="Reset controller", "Message Queue in"=w363) -> ("error out"=w360:errorcluster)  [unwired: 7 in, 1 out]
              }
            }
          }
          event User Event {
            # "Another Module called the \"Find instruments\" API Method."
            n491 = event-data() -> ("Module ID"=w367:i32, "Wait Notifier"=w365:refnum<notifier>, "wait for reply"=w364:bool)  [unwired: 1 in]
            n492 = Bundle(cluster=T25 {"Module ID"=-1, "Wait Notifier"=refnum, "wait for reply"=FALSE} ("Find instruments Argument"), "Module ID"=w367, "Wait Notifier"=w365, "wait for reply"=w364) -> (w368:T25)
            n493 = call "Addressed to This Module.vi"("Module ID from Argument"=w367, "Module Admin"=w370) -> ("Addressed to this instance?"=w371:bool)  [unwired: 8 in, 1 out]
            n494 = case shown="True" w371 {
              tunnel: w372 -> [_ w376]
              tunnel: w368 -> [_ w374]
              tunnel: [_ w373] -> w366
              frame False {
              }
              frame True {
                n495 = call-poly <vilib>:"Delacor_lib_QMH_Enqueue Message (poly).vi"("Message Data"=w374, "Message"="Find instruments", "Message Queue in"=w376) -> ("error out"=w373:errorcluster)  [unwired: 7 in, 1 out]
              }
            }
          }
          event User Event {
            # "Another Module called the \"Connect wihtout dialog\" API Method."
            n496 = event-data() -> ("Module ID"=w380:i32, "VISA resource"=w379:refnum<visa-resource-name>, "baud rate"=w377:u32)  [unwired: 1 in]
            n497 = Bundle(cluster=T26 {"Module ID"=-1, "VISA resource"="", "baud rate"=115200} ("Connect wihtout dialog Argument"), "Module ID"=w380, "VISA resource"=w379, "baud rate"=w377) -> (w381:T26)
            n498 = call "Addressed to This Module.vi"("Module ID from Argument"=w380, "Module Admin"=w383) -> ("Addressed to this instance?"=w384:bool)  [unwired: 8 in, 1 out]
            n499 = case shown="True" w384 {
              tunnel: w385 -> [_ w389]
              tunnel: w381 -> [_ w387]
              tunnel: [_ w386] -> w378
              frame False {
              }
              frame True {
                n500 = call-poly <vilib>:"Delacor_lib_QMH_Enqueue Message (poly).vi"("Message Data"=w387, "Message"="Connect wihtout dialog", "Message Queue in"=w389) -> ("error out"=w386:errorcluster)  [unwired: 7 in, 1 out]
              }
            }
          }
          event User Event {
            # "Another Module called the \"Disconnect\" API Method."
            n501 = event-data() -> ("Module ID"=w392:i32, "Boolean"=w391:bool)  [unwired: 1 in]
            n502 = Bundle(cluster=T27 {"Module ID"=-1, "Boolean"=FALSE} ("Disconnect Argument"), "Module ID"=w392, "Boolean"=w391) -> (w393:T27)
            n503 = call "Addressed to This Module.vi"("Module ID from Argument"=w392, "Module Admin"=w395) -> ("Addressed to this instance?"=w396:bool)  [unwired: 8 in, 1 out]
            n504 = case shown="True" w396 {
              tunnel: w397 -> [_ w401]
              tunnel: w393 -> [_ w399]
              tunnel: [_ w398] -> w390
              frame False {
              }
              frame True {
                n505 = call-poly <vilib>:"Delacor_lib_QMH_Enqueue Message (poly).vi"("Message Data"=w399, "Message"="Disconnect", "Message Queue in"=w401) -> ("error out"=w398:errorcluster)  [unwired: 7 in, 1 out]
              }
            }
          }
          event User Event {
            # "Another Module called the \"Continuously check state\" API Method."
            n506 = event-data() -> ("Module ID"=w406:i32, "Address"=w405:u8, "Desired state"=w404:T1, "Timeout"=w402:i32)  [unwired: 1 in]
            n507 = Bundle(cluster=T28 {"Module ID"=-1, "Address"=0, "Desired state"=enum."Configuration", "Timeout"=0} ("Continuously check state Argument"), "Module ID"=w406, "Address"=w405, "Desired state"=w404, "Timeout"=w402) -> (w407:T28)
            n508 = call "Addressed to This Module.vi"("Module ID from Argument"=w406, "Module Admin"=w409) -> ("Addressed to this instance?"=w410:bool)  [unwired: 8 in, 1 out]
            n509 = case shown="True" w410 {
              tunnel: w411 -> [_ w415]
              tunnel: w407 -> [_ w413]
              tunnel: [_ w412] -> w403
              frame False {
              }
              frame True {
                n510 = call-poly <vilib>:"Delacor_lib_QMH_Enqueue Message (poly).vi"("Message Data"=w413, "Message"="Continuously check state", "Message Queue in"=w415) -> ("error out"=w412:errorcluster)  [unwired: 7 in, 1 out]
              }
            }
          }
          event User Event {
            # "Another Module called the \"Stop checking state\" API Method."
            n511 = event-data() -> ("Module ID"=w418:i32, "Address"=w417:u8)  [unwired: 1 in]
            n512 = Bundle(cluster=T29 {"Module ID"=-1, "Address"=0} ("Stop checking state Argument"), "Module ID"=w418, "Address"=w417) -> (w419:T29)
            n513 = call "Addressed to This Module.vi"("Module ID from Argument"=w418, "Module Admin"=w421) -> ("Addressed to this instance?"=w422:bool)  [unwired: 8 in, 1 out]
            n514 = case shown="True" w422 {
              tunnel: w423 -> [_ w427]
              tunnel: w419 -> [_ w425]
              tunnel: [_ w424] -> w416
              frame False {
              }
              frame True {
                n515 = call-poly <vilib>:"Delacor_lib_QMH_Enqueue Message (poly).vi"("Message Data"=w425, "Message"="Stop checking state", "Message Queue in"=w427) -> ("error out"=w424:errorcluster)  [unwired: 7 in, 1 out]
              }
            }
          }
          event User Event {
            # "Another Module called the \"Configure simultaneous move\" API Method."
            n516 = event-data() -> ("Module ID"=w431:i32, "Address"=w430:u8, "Position"=w429:dbl)  [unwired: 1 in]
            n517 = Bundle(cluster=T30 {"Module ID"=-1, "Address"=0, "Position"=0.0} ("Configure simultaneous move Argument"), "Module ID"=w431, "Address"=w430, "Position"=w429) -> (w432:T30)
            n518 = call "Addressed to This Module.vi"("Module ID from Argument"=w431, "Module Admin"=w434) -> ("Addressed to this instance?"=w435:bool)  [unwired: 8 in, 1 out]
            n519 = case shown="True" w435 {
              tunnel: w436 -> [_ w440]
              tunnel: w432 -> [_ w438]
              tunnel: [_ w437] -> w428
              frame False {
              }
              frame True {
                n520 = call-poly <vilib>:"Delacor_lib_QMH_Enqueue Message (poly).vi"("Message Data"=w438, "Message"="Configure simultaneous move", "Message Queue in"=w440) -> ("error out"=w437:errorcluster)  [unwired: 7 in, 1 out]
              }
            }
          }
          event User Event {
            # "Another Module called the \"Get simultaneous move config\" API Method."
            n521 = event-data() -> ("Module ID"=w445:i32, "Address"=w444:u8, "Wait Notifier"=w443:refnum<notifier>, "wait for reply"=w442:bool)  [unwired: 1 in]
            n522 = Bundle(cluster=T31 {"Module ID"=-1, "Address"=0, "Wait Notifier"=refnum, "wait for reply"=FALSE} ("Get simultaneous move config Argument"), "Module ID"=w445, "Address"=w444, "Wait Notifier"=w443, "wait for reply"=w442) -> (w446:T31)
            n523 = call "Addressed to This Module.vi"("Module ID from Argument"=w445, "Module Admin"=w448) -> ("Addressed to this instance?"=w449:bool)  [unwired: 8 in, 1 out]
            n524 = case shown="True" w449 {
              tunnel: w450 -> [_ w454]
              tunnel: w446 -> [_ w452]
              tunnel: [_ w451] -> w441
              frame False {
              }
              frame True {
                n525 = call-poly <vilib>:"Delacor_lib_QMH_Enqueue Message (poly).vi"("Message Data"=w452, "Message"="Get simultaneous move config", "Message Queue in"=w454) -> ("error out"=w451:errorcluster)  [unwired: 7 in, 1 out]
              }
            }
          }
          event User Event {
            # "Another Module called the \"Execute simultaneous move\" API Method."
            n526 = event-data() -> ("Module ID"=w457:i32, "Boolean"=w456:bool)  [unwired: 1 in]
            n527 = Bundle(cluster=T32 {"Module ID"=-1, "Boolean"=FALSE} ("Execute simultaneous move Argument"), "Module ID"=w457, "Boolean"=w456) -> (w458:T32)
            n528 = call "Addressed to This Module.vi"("Module ID from Argument"=w457, "Module Admin"=w460) -> ("Addressed to this instance?"=w461:bool)  [unwired: 8 in, 1 out]
            n529 = case shown="True" w461 {
              tunnel: w462 -> [_ w466]
              tunnel: w458 -> [_ w464]
              tunnel: [_ w463] -> w455
              frame False {
              }
              frame True {
                n530 = call-poly <vilib>:"Delacor_lib_QMH_Enqueue Message (poly).vi"("Message Data"=w464, "Message"="Execute simultaneous move", "Message Queue in"=w466) -> ("error out"=w463:errorcluster)  [unwired: 7 in, 1 out]
              }
            }
          }
        }
        n531 = call-dynamic "Delacor_lib_QMH_Error Handler - Event Handling Loop.vi"("error in"=w96, "Message Queue in"=w90) -> ("dup error in"=w95:errorcluster)  [unwired: 8 in, 1 out]
      }
      n532 = while {
        tunnel: w34 -> [w51]
        tunnel: [w49] -> w32
        tunnel: w31 -> [w43]
        shift-right: [w48] -> _
        shift-left: -1 -> [w47]
        shift-right: [w46] -> _
        shift-left: T5 {"Instrument Channel"="", "Current state"=enum."Not referenced", "Desired state"=enum."Not referenced", "Address"=1, "Module ID"=0} -> [w45]
        tunnel: [w44] -> w28
        stop <- w50 stop-if-true
        n533 = event shown="[0] Timeout" {
          selector: w51 -> [_ _ _ _]
          dyn-events: [_ _ _ _] -> w49
          timeout: w47 -> [_ _ _ _]
          tunnel: [_ TRUE _ _] -> w50
          tunnel: [w64 w78 w87 -1 ("Timeout")] -> w48
          tunnel: w47 -> [w64 _ _ _]
          tunnel: [w60 w77 w81 w88] -> w46
          tunnel: w45 -> [w61 w77 _ w88]
          tunnel: [w57 _ _ _] -> w44
          tunnel: w43 -> [w55 _ _ _]
          event Timeout {
            n534 = event-data() -> ()  [unwired: 1 in, 1 out]
            n535 = Unbundle By Name(w61) -> ("Module ID"=w56:i32, "Instrument Channel"=w63:string, "Current state"=w62:T1, "Address"=w53:u8, "Desired state"=w52:T1)
            n536 = call "Get state -- subVI.vi"("Instrument Channel"=w63, "Address"=w53, "Device state in"=w62) -> ("error out"=w58:errorcluster, "Device state out"=w54:T1)  [unwired: 7 in]
            n537 = Bundle By Name(cluster=w61, "Current state"=w54) -> (w60:T5)
            n538 = Equal?(x=w54, y=w52) -> (x = y?=w59:bool)
            n539 = case shown="True" w59 {
              tunnel: w58 -> [_ w76]
              tunnel: [_ w73] -> w57
              tunnel: w56 -> [_ w75]
              tunnel: w55 -> [_ w72]
              tunnel: w53 -> [_ w66]
              tunnel: w54 -> [_ w68]
              tunnel: w52 -> [_ w65]
              frame False {
              }
              frame True {
                w67 = T2 {"Address"=0, "Device state out"=enum."Not referenced"}
                n540 = call "State reached.vi"("error in"=w76, "State"=w65, "Address"=w66, "Module ID"=w75) -> ("error out"=w74:errorcluster)  [unwired: 7 in]
                n541 = Bundle By Name(cluster=w67, "Address"=w66, "Device state out"=w68) -> (w69:T2)
                n542 = Build Array(w67, w69) -> (w70:T2[])
                n543 = call-poly <vilib>:"Delacor_lib_QMH_Enqueue Message (poly).vi"("error in"=w74, "Message Data Array"=w70, "Message Array"=string[] ["Stop checking state", "Update state"] ("Message"), "Message Queue in"=w72) -> ("error out"=w73:errorcluster)  [unwired: 6 in, 1 out]
              }
            }
          }
          event User Event {
            w78 = -1  # Timeout
            n544 = event-data() -> ()  [unwired: 1 in, 1 out]
          }
          event User Event {
            n545 = event-data() -> ("Timeout"=w87:i32, "Instrument Channel"=w85:string, "Current state"=w84:T1, "Desired state"=w83:T1, "Address"=w82:u8, "Module ID"=w80:i32)  [unwired: 1 in]
            n546 = Bundle By Name(cluster=T5 {"Instrument Channel"="", "Current state"=enum."Not referenced", "Desired state"=enum."Not referenced", "Address"=1, "Module ID"=0}, "Instrument Channel"=w85, "Current state"=w84, "Desired state"=w83, "Address"=w82, "Module ID"=w80) -> (w81:T5)
          }
          event User Event {
            n547 = event-data() -> ()  [unwired: 1 in, 2 out]
          }
        }
      }
    }
    frame Error {
      n548 = call "Synchronize Caller Events.vi"("Module Admin"=w1400) -> ("Module Admin out"=w1399:refnum<class "Delacor_lib_QMH_Cloneable Module Admin.lvclass">)  [unwired: 9 in, 1 out]
      n549 = property on="Property Node" class="Mod Admin"(reference=w1399) -> ("Accessors:Module ID"=w1398:i32)  [unwired: 1 in, 2 out]
      n550 = call-dynamic "Delacor_lib_QMH_Release Message Queue.vi"("error in"=w1397, "Message Queue"=w1395) -> ("error out"=w1396:errorcluster)  [unwired: 9 in]
      n551 = call "Module Name--constant.vi"("Module ID"=w1398) -> ("Module Name"=w1403:string)  [unwired: 10 in]
      n552 = Format Into String(format string="An error occurred during initialization. %s is no longer running.", w1403) -> (resulting string=w1401:string)  [unwired: 2 in, 1 out]
      n553 = call "Error Reported.vi"("Additional Information"=w1401, "Error"=w1396, "Module ID"=w1398) -> ()  [unwired: 8 in, 1 out]
    }
  }
  n554 = Merge Errors(w26, w25, w3) -> (w27:errorcluster)
  n555 = call "Close Module.vi"("error in"=w27, "Wait for stop?"=w13, "Module Admin in"=w15) -> ("error out"=w23:errorcluster, "External Launch"=w12:bool, "Module Admin out"=w14:refnum<class "Delacor_lib_QMH_Cloneable Module Admin.lvclass">)  [unwired: 6 in]
  n556 = Unregister For Events(event registration refnum=w19, error in=w23) -> (error out=w6:errorcluster)
  n557 = Unregister For Events(event registration refnum=w4, error in=w6) -> (error out=w5:errorcluster)
  "error out" <- w5
  n558 = Bundle(cluster=T2 {"Address"=0, "Device state out"=enum."Not referenced"}, "Device state out"=Device_state_--_enum."Motion" ("Device state")) -> ()  [unwired: 1 in, 1 out]
  n559 = local write "Module Admin"(w14) -> ()
  n560 = case "External Launch?" shown="True" w12 {
    tunnel: w5 -> [_ w1405]
    frame False {
    }
    frame True {
      n561 = case shown="No Error" w1405 {
        frame No Error {
          n562 = invoke class="VI" method="FP.Close"() -> ()  [unwired: 3 in, 3 out]
        }
        frame Error {
          n563 = invoke class="VI" method="FP.Open"("Activate"=TRUE ("Activate?")) -> ()  [unwired: 4 in, 5 out]
        }
      }
    }
  }
